vi "Ballistics_PBBA.vi"() -> ()   [LabVIEW 2012]
uses:
  <vilib>/Utility/NIReport.llb/NI_report.lvclass
  <vilib>/addons/database/NI_Database_API.lvlib
  <vilib>/addons/database/Connection.llb/Conn Execute.vi
  <vilib>/addons/database/Recordset.llb/Rec Destroy - Connection.vi
  <vilib>/Utility/config.llb/NI_LVConfig.lvlib
  <vilib>/Utility/config.llb/Write Key (I32).vi
  <vilib>/addons/database/Connection.llb/DB Tools Open Connec (String).vi
  <vilib>/addons/database/_DB Variant To Data/Database Variant To Data.xnode
  <vilib>/Analysis/NI_AALBase.lvlib
  <vilib>/Utility/config.llb/Write Key (String).vi
  <vilib>/Utility/NIReport.llb/Append Report Text (str wrap).vi
  <vilib>/Utility/NIReport.llb/Append Text Table to Report (wrap).vi
panel:
  in  "Case Constant 2":bool=TRUE
  in  "Case Constant 1":bool
  in  "Contact Shot Report":bool
  in  "message control":bool=TRUE
  in  "Stop Program":bool
  in  "switch":bool
  out "metric conversion":dbl=0.30480370641307 format="%.5f"
  out "number of completes":i32=3
  out "number of partials":i32=2
  in  "percent warning":dbl=1.0 format="%.2f"
  in  "old shots":T1(array[cluster]) {"Red Vel" format="%.2f"; "Energy Loss (J)" format="%.3e"; "Projectile Mass" format="%.4f"; "Corrected residual" format="%.2f"; "Uncorrected Residual" format="%.2f"; "Corrected Impact" format="%.2f"; "Uncorrected Impact" format="%.2f"; "Shot Angle" max=90 step=1; "SHOT STATUS" items=["Partial", "Complete"]; "IMPACT VELOCITY" min=0.0 max=10000.0 step=0.10000000149011612 format="%.1f"; "Barrel Temperature" format="%.1f"; "Powder Loading" format="%.4f"; "RESIDUAL  VELOCITY" min=0.0 max=10000.0 step=0.10000000149011612 format="%.1f"}
  in  "Version":dbl format="%.2f"
  out "Complete":dbl[](array[numeric]) format="%.2f"
  out "Partial":dbl[](array[numeric]) format="%.2f"
  in  "old drag":bool=TRUE
  out "impact/ID":u32=83886081 format="%.0x"
  out "residual/ID":u32=83951617 format="%.0x"
  out "Red/ID":u32=84017153 format="%.0x"
  out "correction coefficient":dbl format="%.8f"
  out "Corrected Residual":dbl format="%.2f"
  out "Corrected Impact":dbl=44.2924057714593 format="%.2f"
  out "plytypes":u16=1
  in  "Number of Ply Types":i32 min=0 max=20 step=1
  out "factor array":dbl[](array[numeric])=[0.0, 0.0, 0.0, 0.0, 0.0, 0.0, 0.0, 0.0, 0.0, 0.0, 0.0, 0.0, 0.0, 0.0, 0.0, 0.0, 0.0, 0.0252, 0.0, 0.0191, 0.0191, 0.0191, 0.0, 0.0, 0.0441, 0.0, 0.0, 0.0, 0.0, 0.0, 0.0, 0.0, 0.0425, 0.0, 0.0, 0.0131, 0.0, 0.0, 0.0, 0.018, 0.0, 0.0, 0.0, 0.0] format="%.4f"
  in  "reread":bool
  out "Weight Units":string
  out "Distance Units":string
  in  "Add Disclaimer":bool
  in  "Report":bool
  in  "RESET":bool
  in  "Save":bool
  in  "EXIT":bool
  in  "String":string="Ply Data Not Entered"
  in  "Enum":T2(ring)
  in  "Impact/Separation":dbl=4.0 format="%.2f"
  in  "Barrel to Screen Distance":dbl=7.8333 format="%.2f"
  in  "Impac/Target Dist":dbl=7.083333 format="%.2f"
  in  "Residual/Separation":dbl=4.0 format="%.2f"
  in  "Residual/Target Dist":dbl=7.083333 format="%.2f"
  out "Z.M.R.":dbl min=0.0 step=0.1 format="%.1f"
  in  "old threat":u32
  out "Shot Graph":cluster{i32[], sgl[]}[](graph)
  in  "Tab Control":T3(tab)
  out "String 2":string="Ballistic Test Program is now initializing.  This requires 30 seconds.  This message will be removed when the program is                ready to be used.                              NOTICE: After initialization, a test bullet must be fired daily to insure superior quality control"
  out "Corrected Redundant":dbl caption="REDUNDANT VELOCITY" min=0.0 max=10000.0 step=0.10000000149011612 format="%.1f"
  in  "backfacedia":dbl
  in  "backdepth":dbl
  out "% Difference":dbl=0.9916409839420799 format="%.1f"
  out "zmr 2":dbl caption="Z.M.R." format="%.1f"
  out "Pairs":i16 min=0 max=100 step=1
  out "Value":dbl format="%.1f"
  in  "Maximum Deviation":dbl=125.0 min=0.0 max=200.0 step=25.0 format="%.1f"
  in  "B.F.S (mm)":u16
  in  "N.I.J":u16(ring) items=["Not Tested", "PASS", "FAIL"]
  in  "Projectile Mass":dbl=7.1278801000000005 caption="Projectile Mass\n(grams)" min=0.0 step=1.0 format="%.4f"
  out "Residual":dbl=1.0 min=0.0 max=1.0 format="%.5f"
  out "Impact":dbl=1.0 min=0.0 max=1.0 format="%.5f"
  out "Shot":i32
  out "Panel":i32
  in  "Data Source":u16(ring)=2 items=["Simulated", "Radar", "Screens"]
  out "Database Connection":string
  in  "Report Path":path=path "c:/ballistic reports"
  in  "red/speed":dbl caption="REDUNDANT VELOCITY" min=0.0 max=1000000.0 step=0.10000000149011612 format="%.1f"
  out "CURRENT TIME / DATE":string
  in  "Current/residual/speed":dbl min=0.0 max=10000.0 step=0.10000000149011612 format="%.1f"
  in  "Current/sthotstatus":u16(ring) items=["Partial", "Complete"]
  in  "Current/impact/speed":dbl min=0.0 max=10000.0 step=0.10000000149011612 format="%.1f"
  in  "Shot Angle":u16 max=90 step=1
  out "BACKFACE DEPTH":dbl caption="BACKFACE\nDEPTH" min=0.0 max=200.0 step=5.0
  out "BACKFACE DIAMETER":dbl caption="BACKFACE\nDIAMETER" min=0.0 max=100.0 step=5.0
  in  "Drag Corrected":bool=TRUE
  in  "Reject shot":bool
  in  "Accept Data":bool
  in  "Powder Loading":dbl min=0.0 max=100.0 step=0.1 format="%.3f"
  in  "Shot Decription":string
  in  "Barrel Temp":dbl format="%.1f"
  out "SUBMIT DATE/TIME":string
  out "residual/speed":dbl caption="RESIDUAL  VELOCITY" min=0.0 max=10000.0 step=0.10000000149011612 format="%.1f"
  out "SHOT STATUS":u16(ring) items=["Partial", "Complete"]
  out "Impact/speed":dbl caption="IMPACT VELOCITY" min=0.0 max=10000.0 step=0.10000000149011612 format="%.1f"
  in  "Table of Shots":string[][](table) caption="Table"
  in  "RANGE RESET":bool
  in  "Tab Control 2":T4(tab)
  in  "Sample ID":string
  in  "Powder Type":u16(ring) items=["ACCURATE, NO. 2", "ACCURATE, NO.9", "Alliant 2400", "Alliant Herc. Bullseye", "Hercules", "Hi-Skor 700x", "Hi-Skor 800x", "IMR-4198", "IMR-4756", "IMR-4895", "International Clay's", "OTHER", "Power Pistol", "WINCHESTER-231", "WINCHESTER-296", "Winchester Ball"]
  in  "Test Comments":string
  in  "Test Conditions":u32(ring) items=["ACCELERATED AGEING", "CONDITIONED", "Cold", "Dry", "Hot 160 DEG. F", "MOTOR OIL", "WEAPON LUBRICANT", "Wet"]
  in  "ballistician":u16(ring) items=["n.a."]
  in  "Method":u16(ring) items=["CUSUM", "N.I.J.", "Quasi N.I.J.", "V(0)", "V(0) @ 1450", "V(0) @ 1500", "V(0) @ 1550", "V50", "VsVr"]
  in  "Room Temperature":i32
  in  "Room Humidity":i32
  in  "Panel Dimensions":u16(ring) items=["101/4\" X 113/4\"", "12X12", "12x15", "13\"X13\"", "15\" x 18\"", "15X16", "15x15", "15x15", "16X16", "18X18", "20X16", "24 x 24", "26X26", "7.5\" X 7.5\"", "8.5\" X 11\"", "CHEST PLATE", "HELMET", "NOT APPLICABLE", "VEST PANEL"]
  in  "Submitter":u16(ring) items=["other"]
  in  "Panel Backing":u16(ring) items=["Aluminum, 24 ga. (.020,.2024-T3) Witness Plate", "Clay (ROMA Plastilina # 1)", "None", "miscellaneous"]
  in  "Threat 2":u32(ring) items=["110-grain(non-toxic)NYLON, 38 SPECIAL, POLY-TUNGSTEN, 10\" SAMMI TEST BBL.", "115-GRAIN,9mm LUGER,REFERENCE ROUND,.38 caliber chamber,10\" TEST BBL.", "115-GRAIN,9mm LUGER,REFERENCE ROUND,10\", 9mm, TEST BBL.", "115-grain, 9 mm, HI-SHOK JHP, +P+ FEDERAL, 10\" SAMMI TEST BBL.", "115-grain, 9 mm, HI-SHOK JHP, +P+ FEDERAL, 5\" SAMMI TEST BBL.", "115-grain,9mm,SMJ,SVENKA-BULLET,CHILE,S.A. 10\"SAMMI TEST BBL.", "123-grain,7.62mm AK-47            7.62mm SAAMI test bbl.", "124-grain,9mm FMJ Rem.#23558, 10\".357cal.SAAMI test bbl.", "124-grain,9mm,FMJ,Rem.#23558, .38 caliber chamber, 10\"SAAMI test bbl.1/10\" TWIST", "124-grain,9mm,FMJ,Rem.#23558, 10\"SAAMI test bbl.", "124-grain,9mm,FMJ,Rem.#23558, 5\"SAAMI test bbl.", "127-grain,9mm,SXT/Blck Tln, +P+,Win.RA9SXT SAAMI test bbl.", "148 grain 7.62 x 51 mm M80 ball", "148-grain,7.62mm FMJ  M80     7.62mm SAAMI test bbl.", "158-grain,0.357, JSP, Rem.#22487 10\"SAAMI test bbl.", "158-grain,0.357, JSP,SPEER.#4217,10\"SAAMI test bbl.", "158-grain,WIN. 357 MAG, JHP REFERENCE ROUND, 10\" SAMMI TEST BBL.", "16-grain,  saboted RCC,.308cal.SAAMI test bbl.,DC", "166-grain,.30 cal. M2 AP, 7.62mm SAAMI test bbl.", "17-grain,sabot,STANAG 2920, FSP,.308 cal. SAMMI test bbl., DC", "17-grain,sabot.Type 1,FSP,.308cal.SAAMI test bbl.,DC", "17-grain,sabot.Type 2,FSP,.308cal.SAAMI test bbl.,DC", "180-grain,40 cal. S&W, 5\"SAMMI test bbl.", "180-grain,WIN. 308 POWER-POINT REFERENCE ROUND, 308 TEST BBL.", "2-grain, saboted RCC FSP,.223cal.SAAMI test bbl.,DC", "207 grain, FSP, 50 Cal", "240 grain,0.44, SWC Speer #4660 no gc,8\"SAAMI test bbl.", "240-grain,0.44, FMJ Speer #4459, 8\" SAMMI test bbl.", "240-grain,0.44, JSP Speer #4457       8\"SAAMI test bbl.", "240-grain,0.44, SJHP,  REM.  # 23592,   8\"SAAMI test bbl.", "240-grain,0.44, SWC PMC w/Gas Check   8\"SAAMI test bbl.", "240-grain,REM. .44 mag, JSP REFERENCE ROUND, 8\" SAMMI TEST BBL.", "4-grain, saboted RCC FSP ,.223cal.SAAMI test bbl.,DC", "44-grain, 0.30-cal FSP - no sabot", "44-grain, 0.30-cal FSP - no sabot", "44-grain,sabot.      FSP,.458cal.SAAMI test bbl.,DC", "45-grain,JHP(WIN), .223 cal. SAMMI test bbl.", "55-grain, 0.223 M-193 FMJ        .223cal.SAAMI test bbl.", "62-grain, 0.223 M-855 Green Tip  .223cal SAAMI test bbl.", "64-grain,sabot.  RCC,.458cal.SAAMI test bbl.,DC", "85-grain(non-toxic), 38 SPECIAL FRANGIBLE,WIN # RA38DF,10\" SAMMI TEST BBL.", "85-grain(non-toxic), 9mm FRANGIBLE +P+,WIN # RA9DF, 5\" SAMMI TEST BBL.", "85-grain(non-toxic), 9mm FRANGIBLE +P+,WIN # RA9DF,10\" SAMMI TEST BBL.", "85-grain, 7.62mm Tokarev(LEAD CORE-STEEL JACKET,1992)Tokarev SAAMI test bbl."]
  in  "Layers":T5(array[cluster])=[{"Ply Description"=0, "Layer Comments"="", "Number of Plies"=1}] {"Number of Plies" min=0 max=99 step=5; "Ply Description" items=["none"]}
  in  "Fabric Description":string
  out "Total Number of Layers":i32=1 caption="Total Number\nof Layers" min=0 max=100 step=5
  in  "Panel Technician":u16(ring) items=["Not Known", "POINT BLANK", "none"]
  in  "Weight of Panel":dbl format="%.4f"
  in  "Areal density text":string
  in  "Areal Density":dbl format="%.2f"
  in  "Thickness":dbl format="%.2f"
  in  "Manufacturer":u32(ring) caption="Mfr" items=["Point Blank-Marine Interceptor"]
  in  "Type":u16(ring) items=["none"]
  in  "Panel Type":u32(ring) items=["COMPOSITE ARMOR", "FABRIC ARMOR", "HELMET", "LG.RIGHT FRONT VEST PANEL", "N.A."]
  in  "Panel Stitch":u32(ring) items=["CAR ARMOR LAMINATE PANEL", "HARD PANEL", "N.A.", "TEST PANEL/CUSTOM STITCH", "TEST PANEL/NORMAL STITCH", "VEST PANEL/CUSTOM STITCH"]
  in  "Next Shot":bool
  in  "Delete Button":bool
  in  "SHOTS":T1(array[cluster]) {"Red Vel" format="%.1f"; "Energy Loss (J)" format="%.3e"; "Projectile Mass" min=0.0 step=1.0 format="%.4f"; "Corrected residual" format="%.2f"; "Uncorrected Residual" format="%.2f"; "Corrected Impact" format="%.2f"; "Uncorrected Impact" format="%.2f"; "Shot Angle" max=90 step=1; "SHOT STATUS" items=["Partial", "Complete"]; "IMPACT VELOCITY" min=0.0 max=10000.0 step=0.10000000149011612 format="%.1f"; "Barrel Temperature" format="%.1f"; "Powder Loading" format="%.4f"; "RESIDUAL  VELOCITY" min=0.0 max=10000.0 step=0.10000000149011612 format="%.1f"}
  out "Data retrieval":string="\nWORKING"
  out "Actual Number of \nRecords Returned":i32=1001
  in  "latest Date":string="1/1/2100"
  in  "DATE 3":string="1/1/2100"
  in  "DATE 2":string="1/1/1900"
  in  "velocity-loading":bool
  in  "Panel Search":bool
  in  "Earliest Date":string="1/1/1900"
  in  "?":u16=1001 min=1 max=10000 step=100
  out "v50 data 2":string[][](table)
  out "In Control":bool=TRUE caption="Control Status"
  in  "Threat":u16(ring) items=["115-GRAIN,9mm LUGER,REFERENCE ROUND,10\" .38 cal TEST BBL.", "158-grain,WIN. 357 MAG, JHP REFERENCE ROUND, 10\" SAMMI TEST BBL.", "180-grain,WIN. 308 POWER-POINT REFERENCE ROUND, 308 TEST BBL.", "240-grain,REM. .44 mag, JSP REFERENCE ROUND, 8\" SAMMI TEST BBL."]
  in  "Powder":string="bul"
  out "St. Deviation":dbl=31.606020957071 format="%.1f"
  out "Latest Velocity":dbl=1314.9 format="%.1f"
  out "Average Velocity":dbl=1297.749514563107 format="%.1f"
  out "Previous V50 Data":cluster{dbl, dbl, dbl[][]}(graph)={0.0, 1.0, []}
  in  "Threat":string
  out "Velocity  versus Loading":cluster{dbl[], dbl[]}(graph)
  out "v50 data":string[][](table)
  out "Device S/N":string
  in  "DAQ Card":i16=1
  in  "Impact Timer":i16 min=0 max=3 step=1
  in  "Redundant Timer":i16=1 min=0 max=3 step=1
  in  "Residual  Timer":i16=2 min=0 max=3 step=1
  # "NOTE:Number of  plies must be entered in FABRIC INFORMATION to enable saving"
  # "yes"
  # "No"
  # "Yes"
  # "No"
  # "Point Blank Body Armor"
  # "Current Shot Data"
  # "Last Assigned  Number"
  # "V50"
  # "Correction Factor"
  # "Edit any non-date field by placing cursor in field. \n\nProperties not listed are controlled by the current shot, test description or Fabric information.  If the entry is changed for the current shot, then all previous shots are changed"
  # "CUSUM HISTORY"
  # "SHOT DATA"
  # "Max Records Returned\n (up to 10,000)"
  # "Date Range"
  # "(Form: 1/25/2000)"
  # "Date Range"
  # "Begin date"
  # "End Date"
  # "(Form: 1/25/2000)"
  # "End Date"
  # "Begin Date"
  # "Point Blank Body Armor\nBallistics Test Station\n\nVersion 1.00 BETA\n\nSeptember 2006"
  # "For technical support contact\n\nPat Fitzgerald or Mark Hartsky\n\nDuPont Company"
  # "This program is beta software and is based on the Ballistics Test Version 2005 developed internally by DuPont as a research tool for their Spruance Plant Ballistics Lab in Richmond, VA.  \n\nThis new version, adapted for use by DHB Point Blank Body Armor, is modified from its original design and does not depend on safety interlock systems to enable operation of a ballistics test.\n\nDuPont makes no warranties and assumes no liabilities in connection with any use of this program."
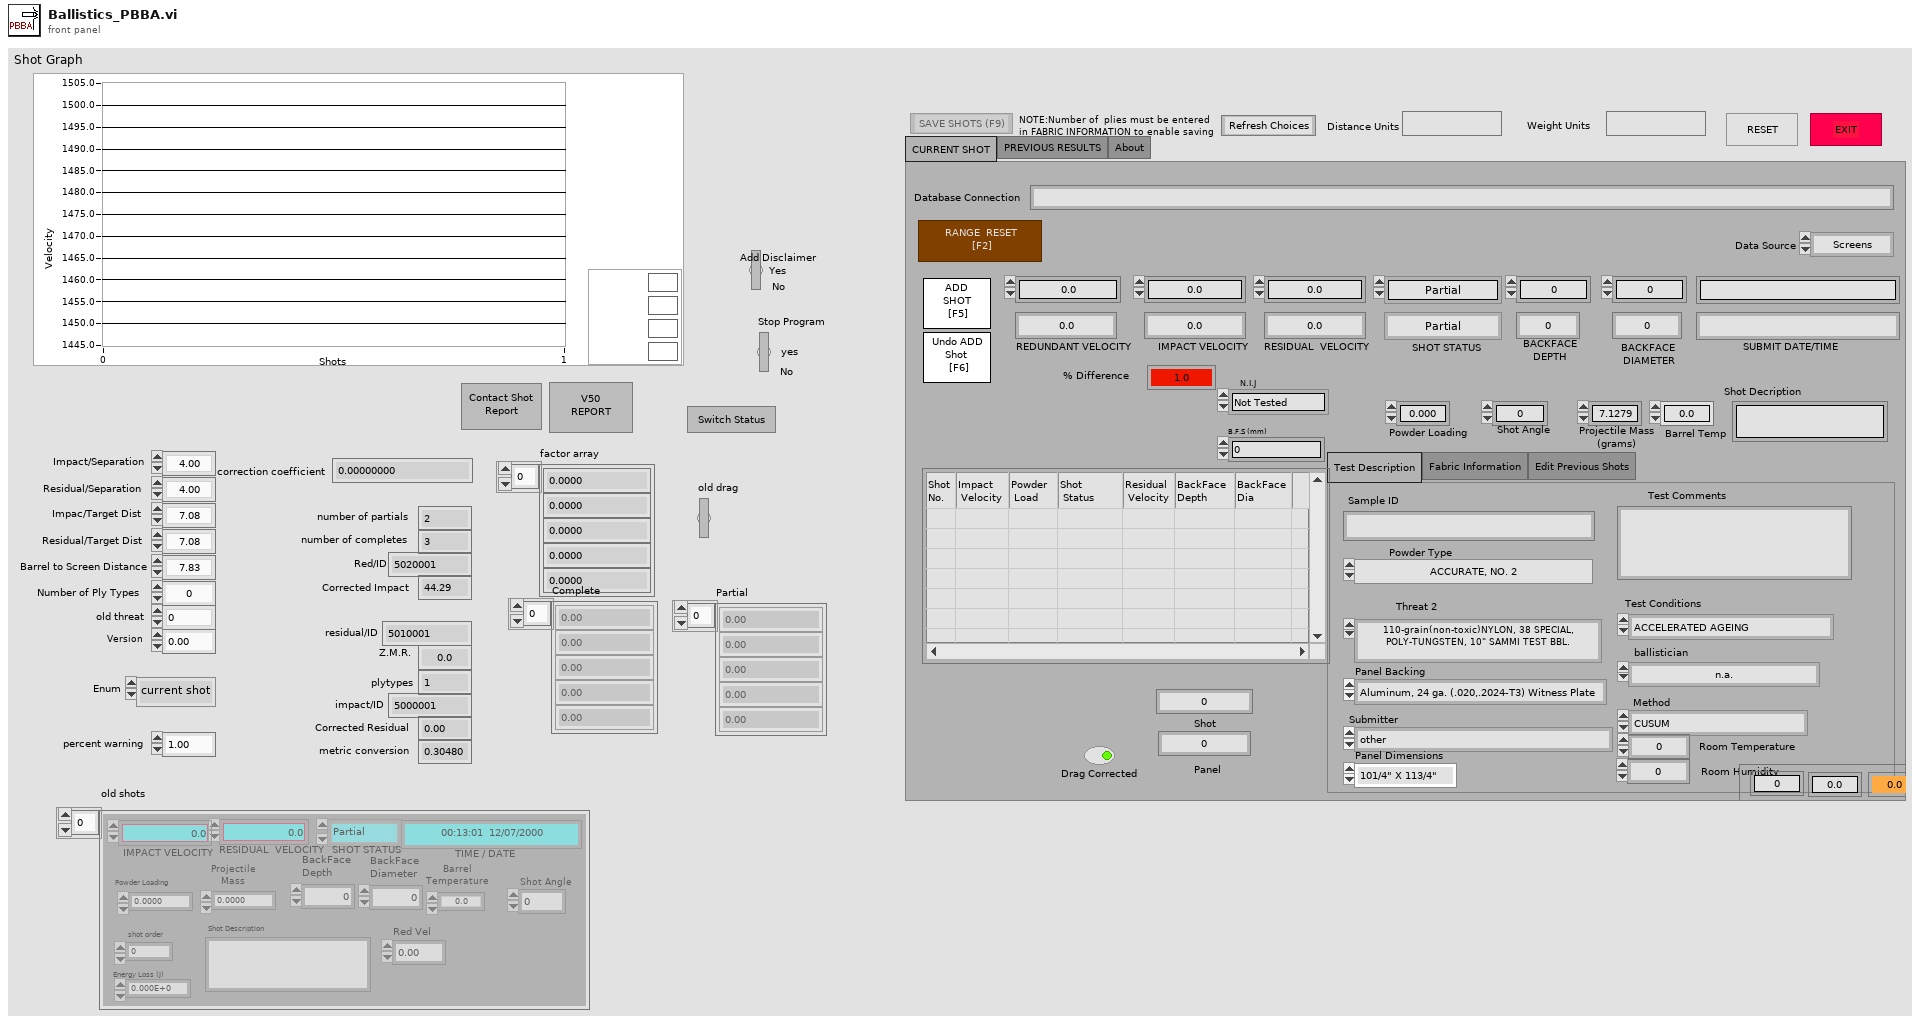
[diagram p1: front panel]
types:
  T1 = cluster{"IMPACT VELOCITY":dbl, "RESIDUAL  VELOCITY ":dbl, "Shot Description":string, "Powder Loading ":dbl, "Barrel Temperature":dbl, "TIME / DATE":string, "shot order":i32, "SHOT STATUS":u16, "Shot Angle":u16, "Uncorrected Impact":dbl, "Corrected Impact":dbl, "Uncorrected Residual":dbl, "Corrected residual":dbl, "Projectile Mass":dbl, "usedv50":bool, "Energy Loss (J)":sgl, "BackFace\nDepth":dbl, "BackFace\nDiameter":dbl, "Red Vel":dbl}[]
  T2 = enum16{"current shot", "previous shots", "controls", "target data"}
  T3 = enum32{"CURRENT SHOT", "PREVIOUS RESULTS", "About"}
  T4 = enum32{"Test Description", "Fabric Information", "Edit Previous Shots"}
  T5 = cluster{"Ply Description":u16, "Layer Comments":string, "Number of Plies":i32}[]
  T6 = cluster{"impactCntrID":u32, "redundantCntrID":u32, "residualCntrID":u32}
  T7 = enum32{"existing file", "new file", "new or existing file", "existing dir", "new dir", "new or existing dir", "existing file (use LLBs)", "new file (use LLBs)", "new or existing file (use LLBs)", "new or existing file or directory (use LLBs)"}
  T8 = typedef "NI_LVConfig.lvlib/Config Data RefNum.ctl" = refnum<k1>
  T9 = cluster{"Charset (-1)":i16, "Weight (-1)":i16, "Name":string, "Size":string}
  T10 = cluster{"Italic":enum16{"Italic Unchanged", "Italic On", "Italic Off"}, "Strike Through":enum16{"Strike Through Unchanged", "Strike Through On", "Strike Through Off"}, "Underline":enum16{"Underline Unchanged", "Underline On", "Underline Off"}, "Bold":enum16{"Bold Unchanged", "Bold On", "Bold Off"}}
  T11 = cluster{"IMPACT VELOCITY":dbl, "RESIDUAL  VELOCITY ":dbl, "Shot Description":string, "Powder Loading ":dbl, "Barrel Temperature":dbl, "TIME / DATE":string, "shot order":i32, "SHOT STATUS":u16, "Shot Angle":u16, "Uncorrected Impact":dbl, "Corrected Impact":dbl, "Uncorrected Residual":dbl, "Corrected residual":dbl, "Projectile Mass":dbl, "usedv50":bool, "Energy Loss (J)":sgl, "BackFace\nDepth":dbl, "BackFace\nDiameter":dbl, "Red Vel":dbl}
  T12 = typedef "NI_Database_API.lvlib/Conn ObjectReference.ctl" = refnum<k1>
  T13 = typedef "NI_Database_API.lvlib/Rec ObjectReference.ctl" = refnum<k1>
  T14 = enum16{"Standard Report", "HTML", "Word", "Excel"}
  T15 = cluster{"task ID out":u32, "task ID out":u32, "task ID out":u32}
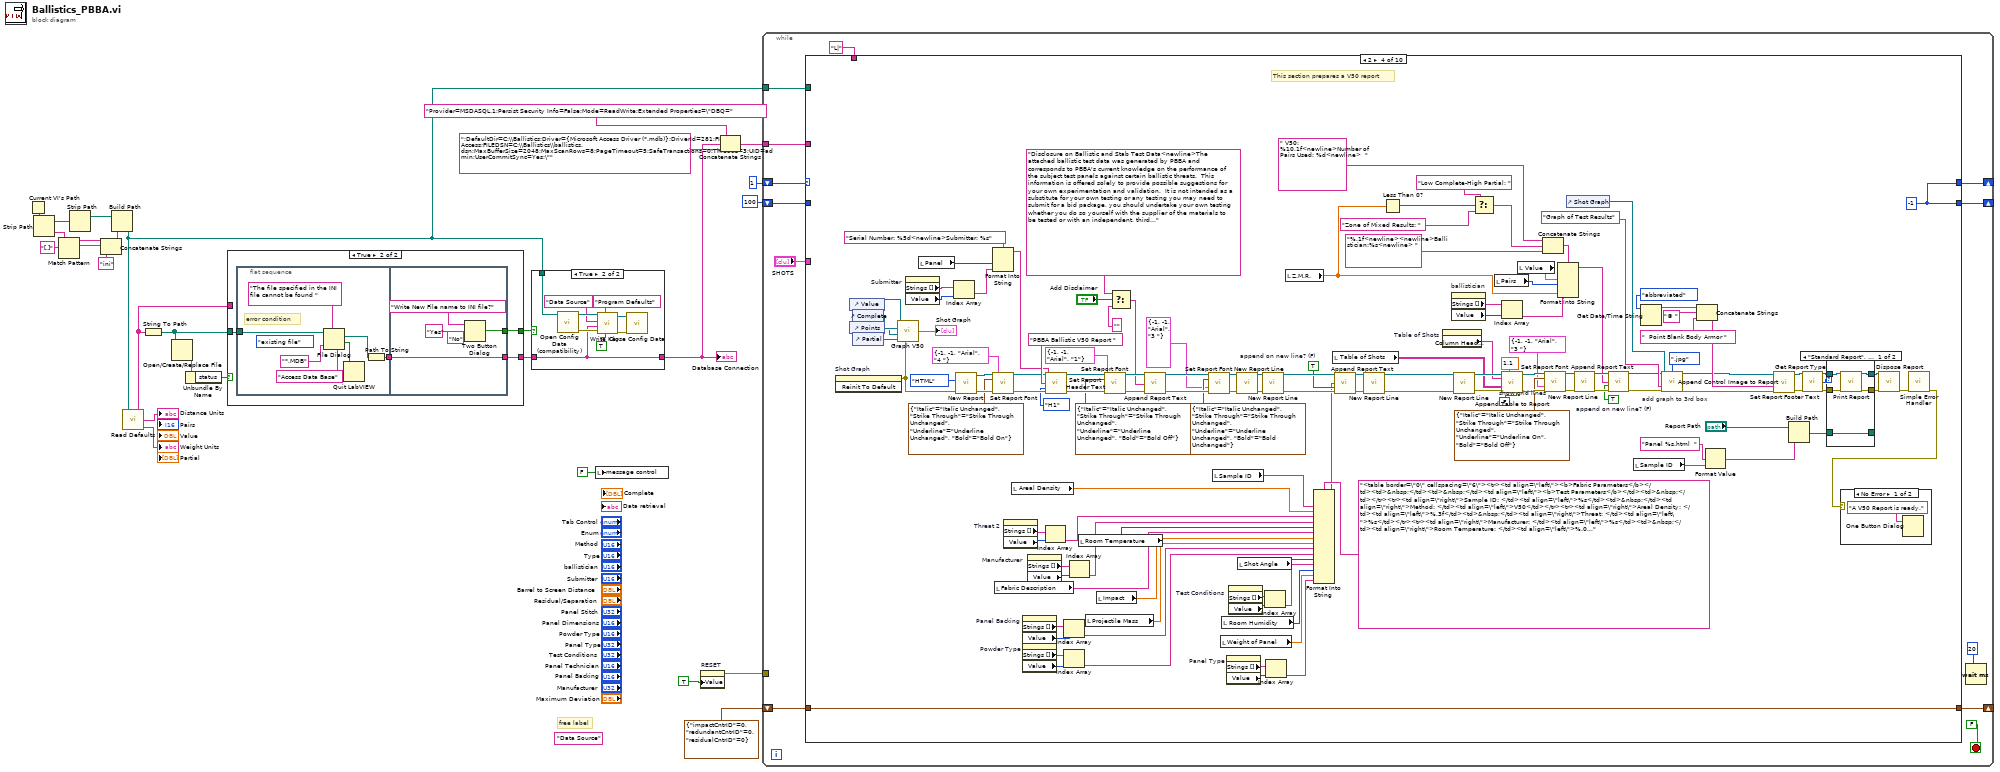
[diagram p0: block diagram]
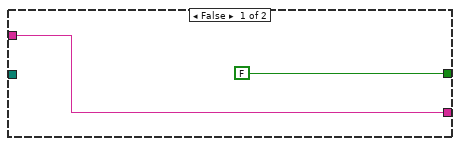
[diagram p3: hidden frame]
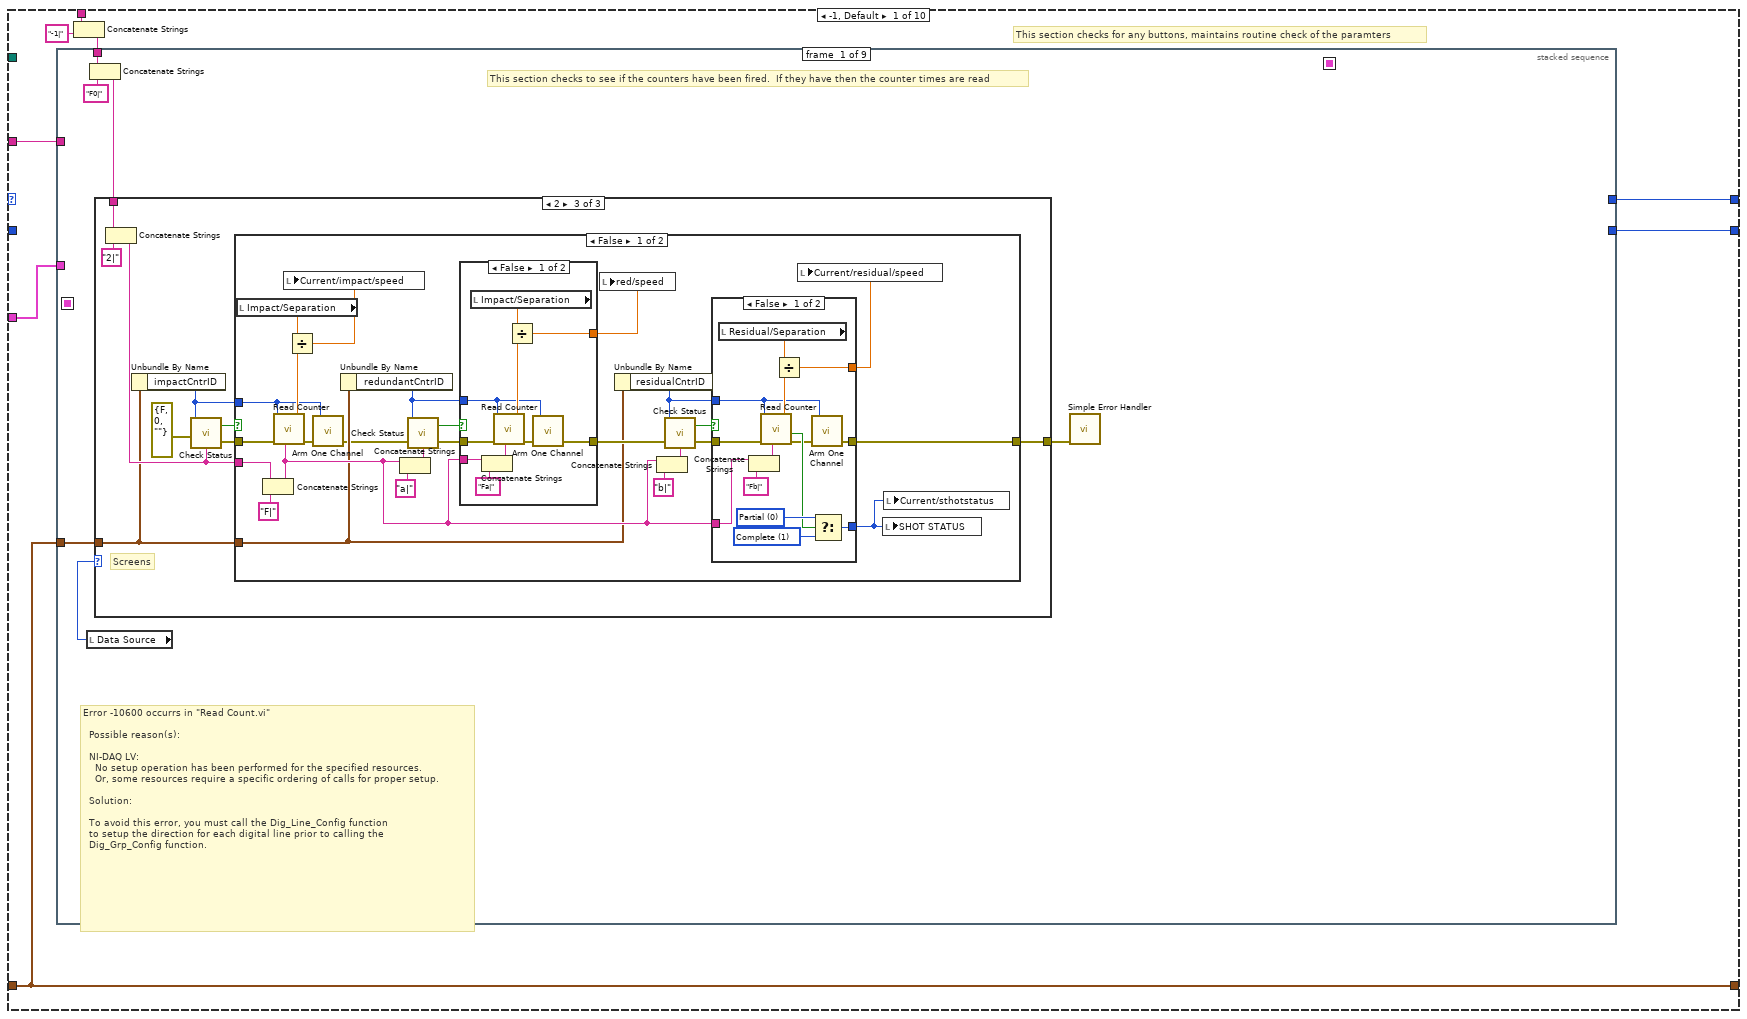
[diagram p4: hidden frame]
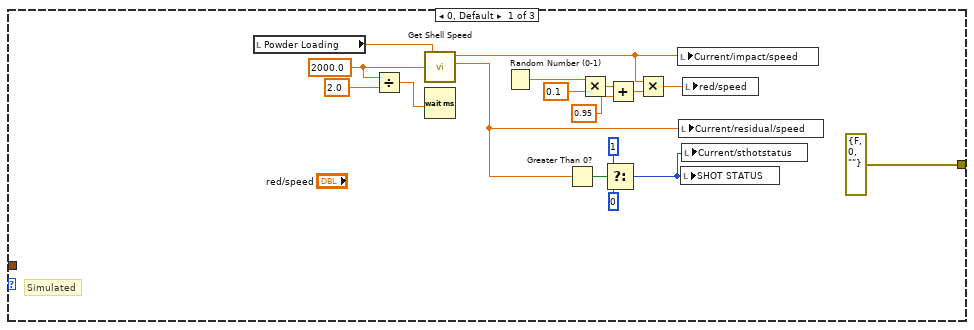
[diagram p5: hidden frame]
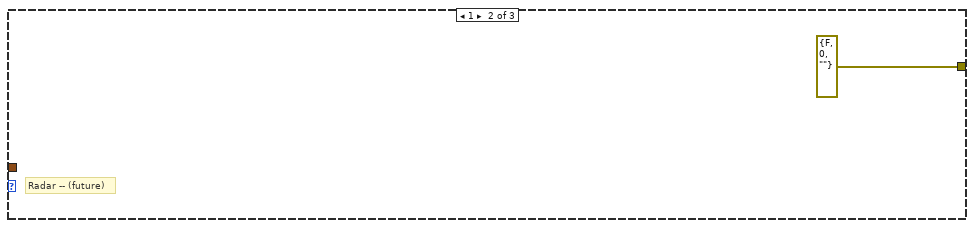
[diagram p6: hidden frame]
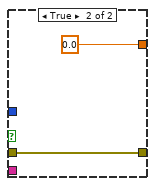
[diagram p7: hidden frame]
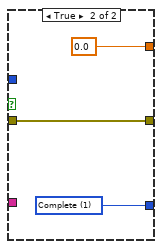
[diagram p8: hidden frame]
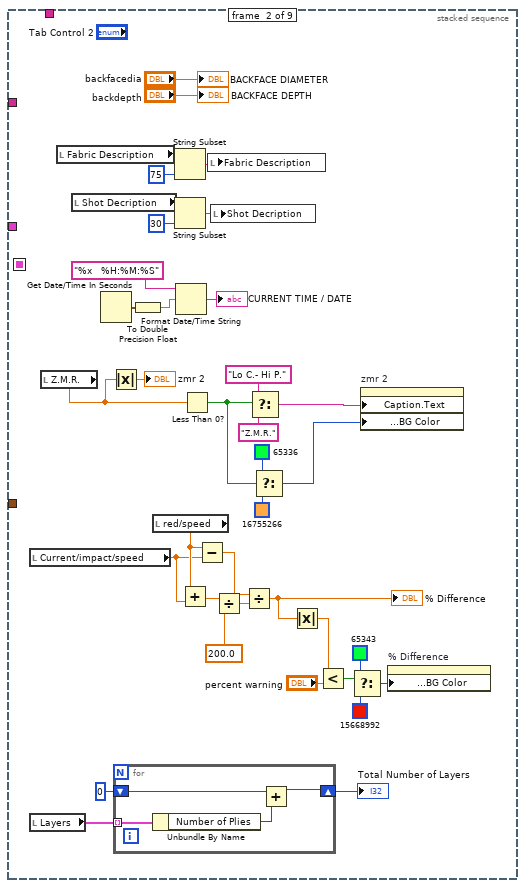
[diagram p10: hidden frame]
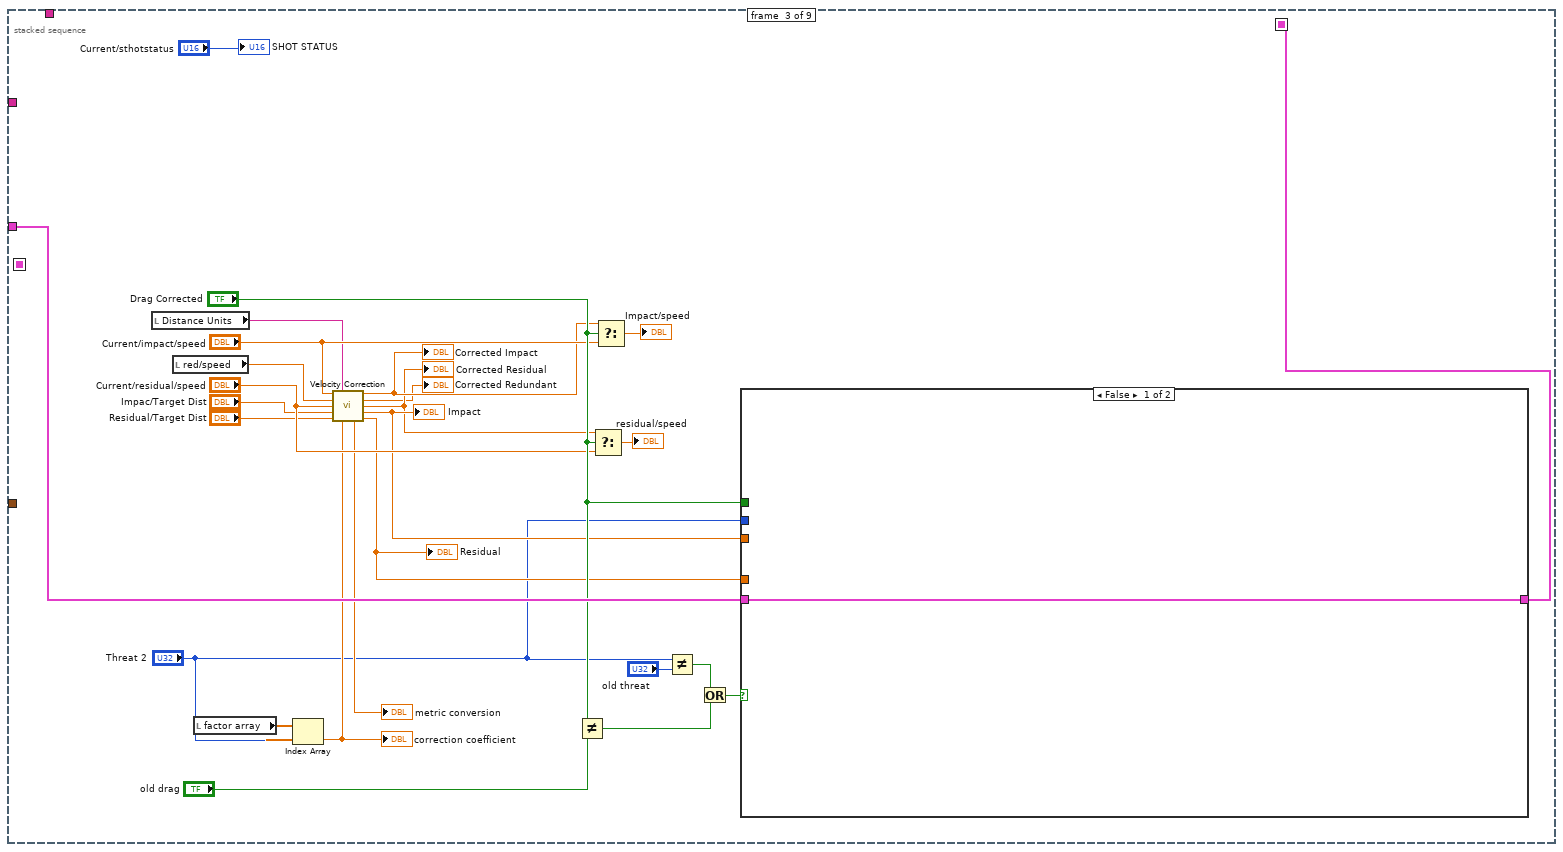
[diagram p11: hidden frame]
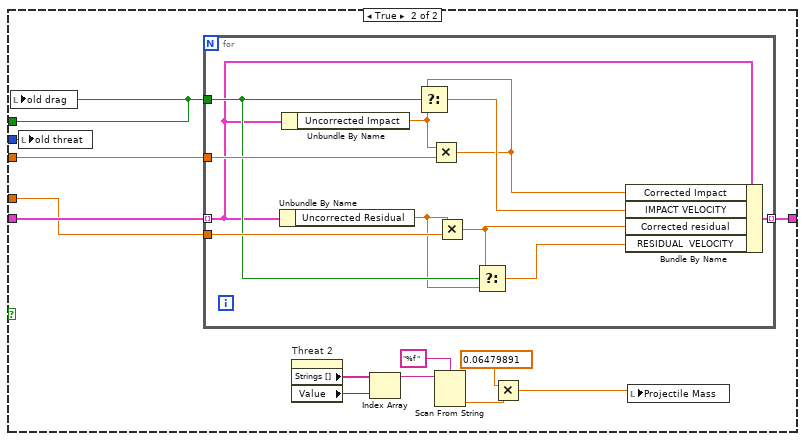
[diagram p12: hidden frame]
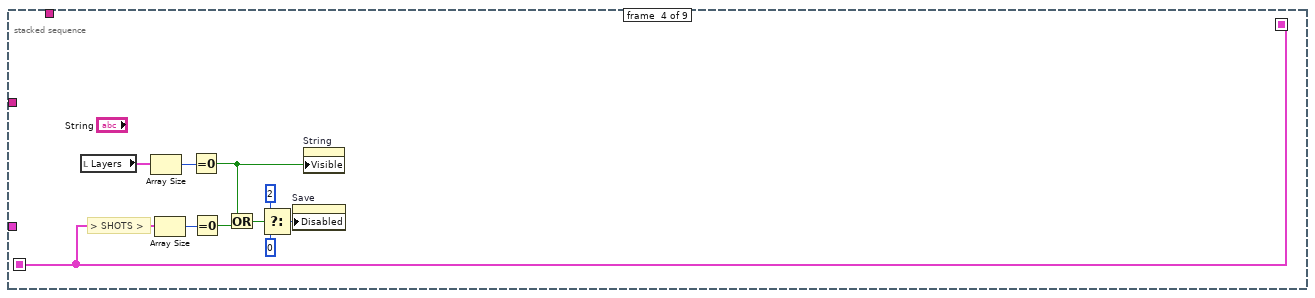
[diagram p13: hidden frame]
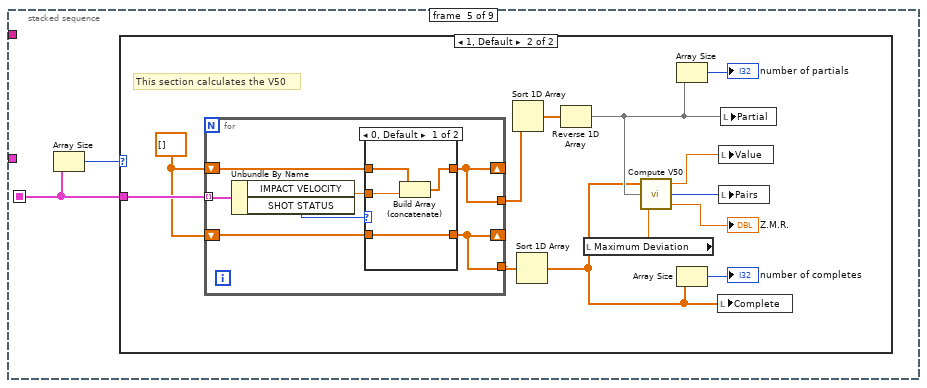
[diagram p14: hidden frame]
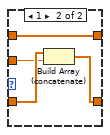
[diagram p16: hidden frame]
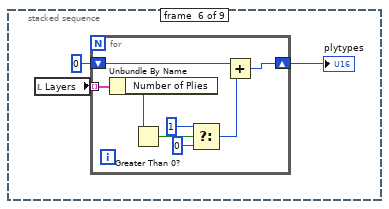
[diagram p17: hidden frame]
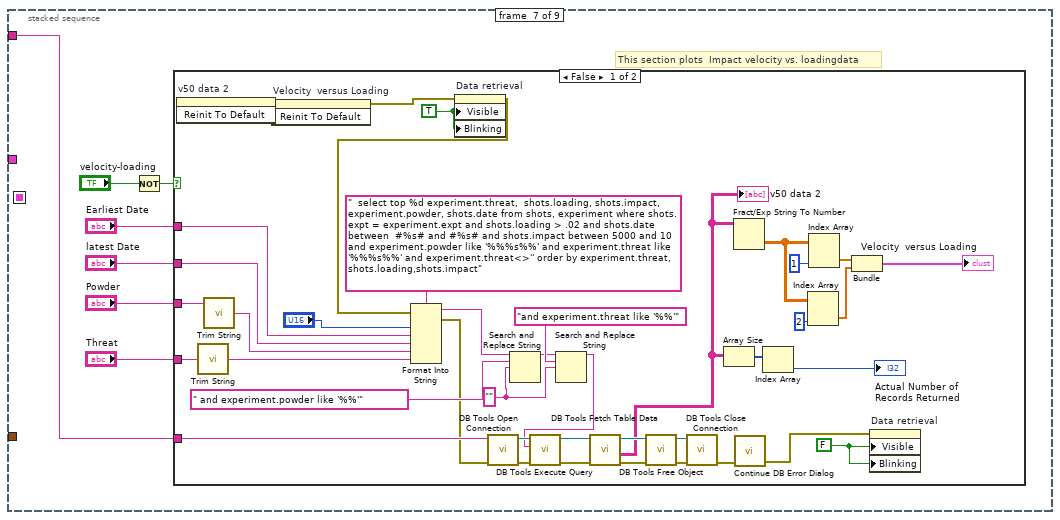
[diagram p18: hidden frame]
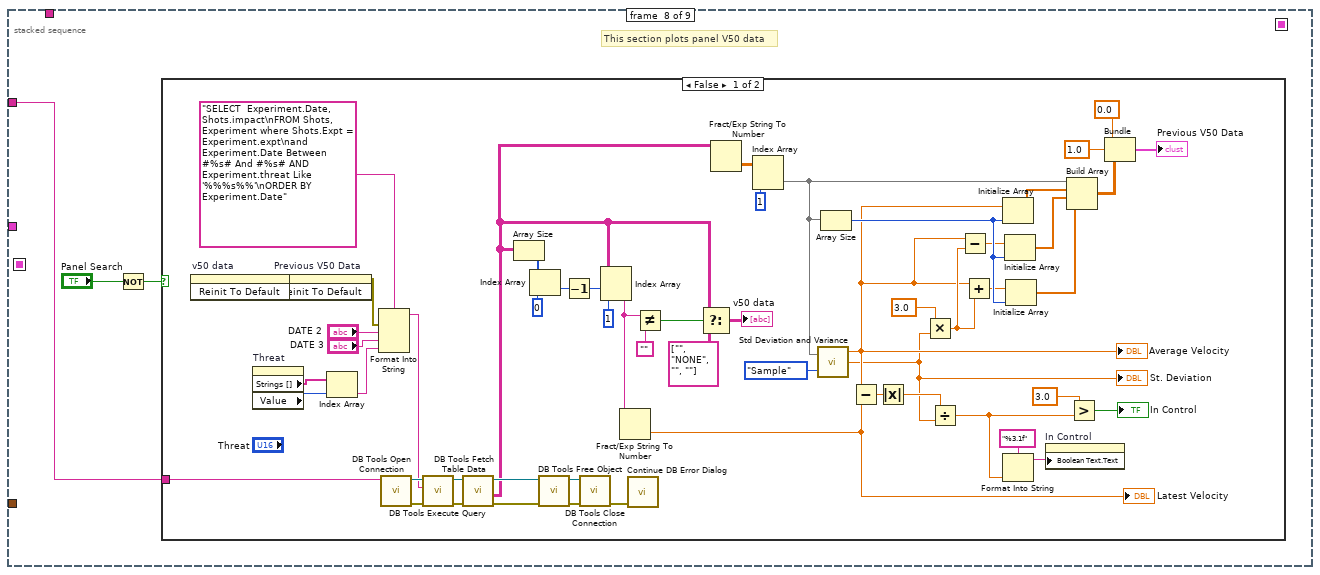
[diagram p20: hidden frame]
diagram:
  (unwired) "Data Source" ("key")
  # "free label"
  n1 = Current VI's Path() -> (path=w25:path)
  n2 = Strip Path(path=w25) -> (stripped path=w24:path, name=w22:string)
  n3 = Match Pattern(string=w22, regular expression="[.]") -> (before substring=w19:string, match substring=w18:string)  [unwired: 1 in, 2 out]
  n4 = Strip Path(path=w24) -> (stripped path=w17:path)  [unwired: 1 out]
  n5 = Concatenate Strings(w19, w18, "ini" ("string")) -> (w21:string)
  n6 = Build Path(base path=w17, name or relative path=w21) -> (appended path=w2:path)
  n7 = call "Read Defaults.vi"("appended path"=w2) -> ("value"=w10:string, "String"=→"Distance Units":string, "String 2"=→"Weight Units":string)
  n8 = String To Path(string=w10) -> (path=w13:path)
  n9 = Open/Create/Replace File(file path (use dialog)=w13) -> (error out=w14:errorcluster)  [unwired: 5 in, 2 out]
  n10 = Unbundle By Name(w14) -> ("status"=w3:bool)
  n11 = case shown="True" w3 {
    tunnel: w10 -> [w30 _]
    tunnel: [w30 w31] -> w9
    tunnel: w13 -> [_ w34]
    tunnel: [FALSE ("T button?") w32] -> w8
    frame False {
    }
    frame True {
      n12 = flat-sequence {
        tunnel: w34 -> [w41]
        tunnel: [w40] -> w33
        tunnel: [w42] -> w31
        tunnel: w33 -> [w42]
        tunnel: [w43] -> w32
        frame #0 {
          (unwired) T7."existing file" ("select mode (2)")
          # "error condition"
          n13 = File Dialog(4:"Access Data Base" ("pattern label"), 6:"*.MDB" ("pattern"), 7:"The file specified in the INI file cannot be found " ("prompt"), 11:w41) -> (1:w35:bool, 3:w38:path)  [unwired: 3 in, 2 out]
          n14 = Quit LabVIEW(quit? (T)=w35) -> ()
          n15 = Path To String(path=w38) -> (string=w40:string)
        }
        frame #1 {
          n16 = Two Button Dialog(message="Write New File name to INI file?", 1:"No" ("F button name (\"Cancel\")"), 2:"Yes" ("T button name (\"OK\")")) -> (T button?=w43:bool)
        }
      }
    }
  }
  n17 = case shown="True" w8 {
    tunnel: w9 -> [w47 w52]
    tunnel: [w47 w52] -> w6
    tunnel: w2 -> [_ w48]
    frame False {
    }
    frame True {
      n18 = call <vilib>:"Open Config Data (compatibility).vi"("configuration file path"=w48) -> ("error out"=w53:errorcluster, "refnum"=w56:T8)  [unwired: 8 in, 1 out]
      n19 = call-poly <vilib>:"Write Key.vi"("write raw string? (F)"=TRUE, "section"="Program Defaults", "error in (no error)"=w53, "value"=w52, "key"="Data Source", "refnum"=w56) -> ("error out"=w51:errorcluster, "refnum out"=w50:T8)  [unwired: 3 in, 1 out]
      n20 = call <vilib>:"Close Config Data.vi"("error in (no error)"=w51, "refnum"=w50) -> ()  [unwired: 8 in, 2 out]
    }
  }
  "Database Connection" <- w6
  n21 = local write "message control"(FALSE) -> ()
  n22 = property on="RESET" class="Bool (strict)"("Value"=TRUE ("RESET")) -> (error out=w4:errorcluster)  [unwired: 2 in, 1 out]
  n23 = Concatenate Strings("Provider=MSDASQL.1;Persist Security Info=False;Mode=ReadWrite;Extended Properties=\"DBQ=", w6, ";DefaultDir=C:\\Ballistics;Driver={Microsoft Access Driver (*.mdb)};DriverId=281;FIL=MS Access;FILEDSN=C:\\Ballistics\\ballistics.dsn;MaxBufferSize=2048;MaxScanRows=8;PageTimeout=5;SafeTransactions=0;Threads=3;UID=admin;UserCommitSync=Yes;\"") -> (w7:string)
  n24 = while {
    shift-left: 100 -> [w64]
    shift-right: [w65] -> _
    shift-left: 1 ("index of element") -> [w68]
    shift-right: [w66] -> _
    tunnel: w2 -> [w61]
    tunnel: w7 -> [w60]
    tunnel: w4 -> [_]
    shift-right: [w58] -> _
    shift-left: T6 {"impactCntrID"=0, "redundantCntrID"=0, "residualCntrID"=0} -> [w57]
    stop <- FALSE stop-if-true
    n25 = case shown="2" w68 {
      tunnel: [w74 w495 w500 w798 w817 w1008 w1046 w1054 w1098 w1221] -> w66
      tunnel: [w75 w495 w500 w798 w816 w1008 w1046 w1054 w1098 w1221] -> w65
      tunnel: w64 -> [_ _ w503 _ _ _ _ _ _ _]
      tunnel: "SHOTS" -> [w76 _ _ _ w815 w998 w1028 _ w1096 _]
      tunnel: w61 -> [_ _ w502 _ w813 _ _ _ _ _]
      tunnel: w60 -> [w73 _ w501 _ w812 _ _ _ _ _]
      tunnel: "L|" -> [w72 _ _ _ _ _ _ w1050 _ _]
      tunnel: [w69 w494 w499 w667 w810 w996 w1011 w1048 w1093 w1149] -> w58
      tunnel: w57 -> [w69 w494 w499 w667 w810 w996 w1011 w1047 w1093 w1149]
      frame -1, Default {
        # "This section checks for any buttons, maintains routine check of the paramters"
        n26 = Concatenate Strings(w72, "-1|") -> (w70:string)
        n27 = stacked-sequence {
          seq-local: [_ _ _ w258 _ _ _ _ _] -> [_ _ _ _ w269 _ _ _ w424]
          seq-local: [_ _ w221 _ _ _ _ _ _] -> [_ _ _ w258 _ _ _ _ _]
          tunnel: w76 -> [_ _ w227 _ _ _ _ _ _]
          tunnel: [_ _ _ _ _ _ _ _ w429] -> w74
          tunnel: [_ _ _ _ _ _ _ _ -1] -> w75
          tunnel: w73 -> [_ _ _ _ _ _ w309 w356 _]
          tunnel: w70 -> [w80 _ _ _ _ _ _ _ _]
          tunnel: w69 -> [w77 _ _ _ _ _ _ _ _]
          frame #0 {
            # "Error -10600 occurrs in \"Read Count.vi\"\n\n  Possible reason(s):\n\n  NI-DAQ LV:\n    No setup operation has been performed for the specified resources.\n    Or, some resources require a specific ordering of calls for proper setup.  \n\n  Solution: \n\n  To avoid this error, you must call the Dig_Line_Config function \n  to setup the direction for each digital line prior to calling the \n  Dig_Grp_Config function."
            # "This section checks to see if the counters have been fired.  If they have then the counter times are read"
            n28 = local read "Data Source"() -> (w82:u16)
            n29 = Concatenate Strings(w80, "F0|") -> (w78:string)
            n30 = case shown="2" w82 {
              tunnel: [errorcluster {"status"=FALSE, "code"=0, "source"=""} ("error out") errorcluster {"status"=FALSE, "code"=0, "source"=""} ("error out") w109] -> w81
              tunnel: w78 -> [_ _ w105]
              tunnel: w77 -> [_ _ w101]
              frame 0, Default {
                w98 = 2000.0 ("v50")
                # "Simulated"
                n31 = local read "Powder Loading"() -> (w97:dbl)
                n32 = Divide(x=w98, y=2.0 ("v50")) -> (x/y=w99:dbl)
                n33 = call "Get Shell Speed.vi"("loading"=w97, "v50"=w98) -> ("impact"=w85:sgl, "residual"=w91:sgl)  [unwired: 2 in, 1 out]
                n34 = Wait (ms)(milliseconds to wait=w99) -> ()  [unwired: 1 out]
                n35 = Random Number (0-1)() -> (number: 0 to 1=w89:dbl)
                n36 = Greater Than 0?(x=w91) -> (x > 0?=w94:bool)
                n37 = Multiply(x=w89, y=0.1) -> (x*y=w88:dbl)
                n38 = Select(t=u16 1, s=w94, f=u16 0) -> (s? t:f=w92:u16)
                n39 = Add(x=w88, y=0.95) -> (x+y=w86:dbl)
                n40 = Multiply(x=w85, y=w86) -> (x*y=w84:dbl)
                n41 = local write "Current/impact/speed"(w85) -> ()
                n42 = local write "Current/residual/speed"(w91) -> ()
                n43 = local write "SHOT STATUS"(w92) -> ()
                n44 = local write "Current/sthotstatus"(w92) -> ()
                n45 = local write "red/speed"(w84) -> ()
              }
              frame 1 {
                # "Radar -- (future)"
              }
              frame 2 {
                # "Screens"
                n46 = Concatenate Strings(w105, "2|") -> (w104:string)
                n47 = Unbundle By Name(w101) -> ("impactCntrID"=w102:u32)
                n48 = call "Check Status.vi"("error in (no error)"=errorcluster {"status"=FALSE, "code"=0, "source"=""}, "TL Calling Location"=w104, "Task ID"=w102) -> ("error out"=w107:errorcluster, "Armed?"=w103:bool)  [unwired: 1 in]
                n49 = case shown="False" w103 {
                  tunnel: w107 -> [w127 w165]
                  tunnel: [w128 w165] -> w109
                  tunnel: w102 -> [w110 _]
                  tunnel: w104 -> [w123 _]
                  tunnel: w101 -> [w113 _]
                  frame False {
                    n50 = local read "Impact/Separation"() -> (w132:dbl)
                    n51 = Concatenate Strings(w123, "F|") -> (w118:string)
                    n52 = call "Read Counter.vi"("TL Calling Location"=w118, "error In"=w127, "TASK ID"=w110) -> ("error out"=w112:errorcluster, "time (secs)"=w135:sgl)  [unwired: 3 in, 2 out]
                    n53 = Divide(x=w132, y=w135) -> (x/y=w130:dbl)
                    n54 = local write "Current/impact/speed"(w130) -> ()
                    n55 = call "Arm One Channel.vi"("error IN"=w112, "task ID IN"=w110) -> ("error out"=w111:errorcluster)  [unwired: 2 in, 1 out]
                    n56 = Unbundle By Name(w113) -> ("redundantCntrID"=w115:u32)
                    n57 = Concatenate Strings(w118, "a|") -> (w121:string)
                    n58 = call "Check Status.vi"("error in (no error)"=w111, "TL Calling Location"=w121, "Task ID"=w115) -> ("error out"=w126:errorcluster, "Armed?"=w117:bool)  [unwired: 1 in]
                    n59 = case shown="False" w117 {
                      tunnel: [w143 0.0] -> w134
                      tunnel: w126 -> [w142 w147]
                      tunnel: [w137 w147] -> w129
                      tunnel: w115 -> [w136 _]
                      tunnel: w118 -> [w140 _]
                      frame False {
                        n60 = local read "Impact/Separation"() -> (w144:dbl)
                        n61 = Concatenate Strings(w140, "Fa|") -> (w139:string)
                        n62 = call "Read Counter.vi"("TL Calling Location"=w139, "error In"=w142, "TASK ID"=w136) -> ("error out"=w138:errorcluster, "time (secs)"=w145:sgl)  [unwired: 3 in, 2 out]
                        n63 = Divide(x=w144, y=w145) -> (x/y=w143:dbl)
                        n64 = call "Arm One Channel.vi"("error IN"=w138, "task ID IN"=w136) -> ("error out"=w137:errorcluster)  [unwired: 2 in, 1 out]
                      }
                      frame True {
                      }
                    }
                    n65 = local write "red/speed"(w134) -> ()
                    n66 = Unbundle By Name(w113) -> ("residualCntrID"=w114:u32)
                    n67 = Concatenate Strings(w118, "b|") -> (w119:string)
                    n68 = call "Check Status.vi"("error in (no error)"=w129, "TL Calling Location"=w119, "Task ID"=w114) -> ("error out"=w125:errorcluster, "Armed?"=w116:bool)  [unwired: 1 in]
                    n69 = case shown="False" w116 {
                      tunnel: w125 -> [w154 w163]
                      tunnel: [w159 w164] -> w133
                      tunnel: w114 -> [w149 _]
                      tunnel: [w148 w163] -> w128
                      tunnel: [w156 0.0] -> w131
                      tunnel: w118 -> [w151 _]
                      frame False {
                        w160 = u16 1 items=["Partial", "Complete"] ("SHOT STATUS")
                        w161 = u16 0 items=["Partial", "Complete"] ("SHOT STATUS")
                        n70 = local read "Residual/Separation"() -> (w155:dbl)
                        n71 = Concatenate Strings(w151, "Fb|") -> (w152:string)
                        n72 = call "Read Counter.vi"("TL Calling Location"=w152, "error In"=w154, "TASK ID"=w149) -> ("error out"=w150:errorcluster, "counter overflow?"=w157:bool, "time (secs)"=w158:sgl)  [unwired: 3 in, 1 out]
                        n73 = Divide(x=w155, y=w158) -> (x/y=w156:dbl)
                        n74 = call "Arm One Channel.vi"("error IN"=w150, "task ID IN"=w149) -> ("error out"=w148:errorcluster)  [unwired: 2 in, 1 out]
                        n75 = Select(t=w161, s=w157, f=w160) -> (s? t:f=w159:u16)
                      }
                      frame True {
                        (unwired) 0.0
                        w164 = u16 1 items=["Partial", "Complete"] ("SHOT STATUS")
                      }
                    }
                    n76 = local write "Current/residual/speed"(w131) -> ()
                    n77 = local write "SHOT STATUS"(w133) -> ()
                    n78 = local write "Current/sthotstatus"(w133) -> ()
                  }
                  frame True {
                  }
                }
              }
            }
            n79 = call <vilib>:"Simple Error Handler.vi"("error in (no error)"=w81) -> ()  [unwired: 4 in, 5 out]
          }
          frame #1 {
            n80 = local read "Current/impact/speed"() -> (w185:dbl)
            n81 = local read "Layers"() -> (w201:T5)
            n82 = local read "Z.M.R."() -> (w188:dbl)
            n83 = local read "Fabric Description"() -> (w172:string)
            n84 = local read "Shot Decription"() -> (w169:string)
            n85 = Get Date/Time In Seconds() -> (seconds since 1Jan1904=w166:timestamp)
            n86 = Absolute Value(x=w188) -> (abs(x)=→"zmr 2":dbl)
            n87 = for {
              tunnel: w201 -> [w203] mode=indexing
              shift-right: [w205] -> w199
              shift-left: 0 -> [w204]
              n88 = Unbundle By Name(w203) -> ("Number of Plies"=w206:i32)
              n89 = Add(x=w204, y=w206) -> (x+y=w205:i32)
            }
            "Total Number of Layers" <- w199
            n90 = To Double Precision Float(number=w166) -> (double precision float=w196:dbl)
            n91 = local read "red/speed"() -> (w186:dbl)
            n92 = String Subset(string=w172, length (rest)=75 ("length (rest)")) -> (substring=w171:string)  [unwired: 1 in]
            n93 = String Subset(string=w169, length (rest)=30 ("length (rest)")) -> (substring=w167:string)  [unwired: 1 in]
            n94 = Format Date/Time String(time format string (%c)="%x   %H:%M:%S", seconds (now)=w196) -> (date/time string=→"CURRENT TIME / DATE":string)  [unwired: 1 in]
            n95 = Add(x=w186, y=w185) -> (x+y=w184:dbl)
            n96 = Less Than 0?(x=w188) -> (x < 0?=w194:bool)
            n97 = Subtract(x=w186, y=w185) -> (x-y=w187:dbl)
            n98 = local write "Fabric Description"(w171) -> ()
            n99 = local write "Shot Decription"(w167) -> ()
            n100 = Divide(x=w184, y=200.0) -> (x/y=w183:dbl)
            n101 = Divide(x=w187, y=w183) -> (x/y=w179:dbl)
            "% Difference" <- w179
            n102 = Select(t="Lo C.- Hi P.", s=w194, f="Z.M.R.") -> (s? t:f=w191:string)
            n103 = Select(t=u32 65336, s=w194, f=u32 16755266) -> (s? t:f=w190:u32)
            n104 = Absolute Value(x=w179) -> (abs(x)=w176:dbl)
            n105 = Less?(x=w176, y="percent warning") -> (x < y?=w177:bool)
            n106 = Select(t=u32 65343, s=w177, f=u32 15668992) -> (s? t:f=w175:u32)
            n107 = property on="zmr 2" class="DigNum (strict)"("Caption.Text"=w191, "Numeric Text.Text Colors:BG Color"=w190) -> ()  [unwired: 2 in, 2 out]
            n108 = property on="% Difference" class="DigNum (strict)"("Numeric Text.Text Colors:BG Color"=w175) -> ()  [unwired: 2 in, 2 out]
            "BACKFACE DIAMETER" <- "backfacedia"
            "BACKFACE DEPTH" <- "backdepth"
          }
          frame #2 {
            n109 = local read "Distance Units"() -> (w219:string)
            n110 = local read "red/speed"() -> (w218:dbl)
            n111 = local read "factor array"() -> (w231:dbl[])
            n112 = Index Array(array=w231, index="Threat 2") -> (element=w213:dbl)
            "correction coefficient" <- w213
            n113 = call "Velocity Correction.vi"("raw impact"="Current/impact/speed", "distance units"=w219, "raw redundant"=w218, "raw residual"="Current/residual/speed", "screen set midpt to target"="Impac/Target Dist", "residual screen to target"="Residual/Target Dist", "correction coefficient"=w213) -> ("corrected impact"=w214:sgl, "corrected redundant"=→"Corrected Redundant":sgl, "corrected residual"=w209:sgl, "impact factor"=w210:sgl, "conversion factor"=→"metric conversion":sgl, "residual factor"=w211:sgl)  [unwired: 3 in]
            "Residual" <- w211
            "Impact" <- w210
            "Corrected Impact" <- w214
            "Corrected Residual" <- w209
            n114 = Not Equal?(x="Drag Corrected", y="old drag") -> (x != y?=w223:bool)
            n115 = Select(t=w209, s="Drag Corrected", f="Current/residual/speed") -> (s? t:f=→"residual/speed":dbl)
            n116 = Select(t=w214, s="Drag Corrected", f="Current/impact/speed") -> (s? t:f=→"Impact/speed":dbl)
            n117 = Not Equal?(x="Threat 2", y="old threat") -> (x != y?=w224:bool)
            n118 = Or(x=w224, y=w223) -> (x .or. y?=w222:bool)
            n119 = case shown="False" w222 {
              tunnel: "Threat 2" -> [_ w246]
              tunnel: w227 -> [w233 w245]
              tunnel: w211 -> [_ w244]
              tunnel: w210 -> [_ w243]
              tunnel: "Drag Corrected" -> [_ w242]
              tunnel: [w233 w241] -> w221
              frame False {
              }
              frame True {
                n120 = local write "old drag"(w242) -> ()
                n121 = local write "old threat"(w246) -> ()
                n122 = for {
                  tunnel: w245 -> [w249] mode=indexing
                  tunnel: w244 -> [w257]
                  tunnel: w243 -> [w256]
                  tunnel: w242 -> [w253]
                  tunnel: [w251] -> w241 mode=indexing
                  n123 = Unbundle By Name(w249) -> ("Uncorrected Residual"=w250:dbl)
                  n124 = Unbundle By Name(w249) -> ("Uncorrected Impact"=w255:dbl)
                  n125 = Multiply(x=w255, y=w256) -> (x*y=w248:dbl)
                  n126 = Select(t=w248, s=w253, f=w255) -> (s? t:f=w252:dbl)
                  n127 = Multiply(x=w250, y=w257) -> (x*y=w254:dbl)
                  n128 = Select(t=w254, s=w253, f=w250) -> (s? t:f=w247:dbl)
                  n129 = Bundle By Name(cluster=w249, "Corrected Impact"=w248, "IMPACT VELOCITY"=w252, "Corrected residual"=w254, "RESIDUAL  VELOCITY"=w247) -> (w251:T11)
                }
                n130 = property on="Threat 2" class="Ring (strict)"() -> ("Strings []"=w240:string[], "Value"=w239:u32)  [unwired: 2 in, 2 out]
                n131 = Index Array(array=w240, index=w239) -> (element=w238:string)
                n132 = Scan From String(format string="%f " ("Format String"), input string=w238) -> (output 1=w236:dbl)  [unwired: 3 in, 3 out]
                n133 = Multiply(x=0.06479891, y=w236) -> (x*y=w234:dbl)
                n134 = local write "Projectile Mass"(w234) -> ()
              }
            }
            "SHOT STATUS" <- "Current/sthotstatus"
          }
          frame #3 {
            # "> SHOTS >"
            n135 = local read "Layers"() -> (w261:T5)
            n136 = Array Size(array=w261) -> (size(s)=w260:i32)
            n137 = Array Size(array=w258) -> (size(s)=w267:i32)
            n138 = Equal To 0?(x=w260) -> (x = 0?=w266:bool)
            n139 = Equal To 0?(x=w267) -> (x = 0?=w265:bool)
            n140 = Or(x=w266, y=w265) -> (x .or. y?=w264:bool)
            n141 = Select(t=u8 2, s=w264, f=u8 0) -> (s? t:f=w259:u8)
            n142 = property on="Save" class="Bool"("Disabled"=w259) -> ()  [unwired: 2 in, 2 out]
            n143 = property on="String" class="Str"("Visible"=w266) -> ()  [unwired: 2 in, 2 out]
          }
          frame #4 {
            n144 = Array Size(array=w269) -> (size(s)=w268:i32)
            n145 = case shown="1, Default" w268 {
              tunnel: w269 -> [_ w272]
              frame 0 {
              }
              frame 1, Default {
                w270 = dbl[] [] ("Partial")
                # "This section calculates the V50"
                n146 = for {
                  tunnel: [w287] -> w281
                  shift-right: [w287] -> _
                  shift-left: w270 -> [w288]
                  shift-right: [w285] -> _
                  shift-left: w270 -> [w286]
                  tunnel: [w285] -> w282
                  tunnel: w272 -> [w284] mode=indexing
                  n147 = Unbundle By Name(w284) -> ("IMPACT VELOCITY"=w289:dbl, "SHOT STATUS"=w283:u16)
                  n148 = case shown="0, Default" w283 {
                    tunnel: w289 -> [w290 w294]
                    tunnel: [w293 w295] -> w287
                    tunnel: w288 -> [w292 w295]
                    tunnel: w286 -> [w291 w297]
                    tunnel: [w291 w296] -> w285
                    frame 0, Default {
                      n149 = Build Array (concatenate)(w292, w290) -> (w293:dbl[])
                    }
                    frame 1 {
                      n150 = Build Array (concatenate)(w297, w294) -> (w296:dbl[])
                    }
                  }
                }
                n151 = Sort 1D Array(array=w281) -> (sorted array=w280:dbl[])
                n152 = Sort 1D Array(array=w282) -> (sorted array=w273:dbl[])
                n153 = Reverse 1D Array(array=w280) -> (reversed array=w276:dbl[])
                n154 = local read "Maximum Deviation"() -> (w279:dbl)
                n155 = call "Compute V50.vi"("Maximum Deviation"=w279, "Partial"=w276, "Complete"=w273) -> ("zmr"=→"Z.M.R.":sgl, "Points"=w277:i16, "V50"=w271:sgl)
                n156 = Array Size(array=w276) -> (size(s)=→"number of partials":i32)
                n157 = Array Size(array=w273) -> (size(s)=→"number of completes":i32)
                n158 = local write "Complete"(w273) -> ()
                n159 = local write "Value"(w271) -> ()
                n160 = local write "Pairs"(w277) -> ()
                n161 = local write "Partial"(w276) -> ()
              }
            }
          }
          frame #5 {
            n162 = local read "Layers"() -> (w300:T5)
            n163 = for {
              tunnel: w300 -> [w308] mode=indexing
              shift-right: [w305] -> w299
              shift-left: u16 0 -> [w306]
              n164 = Unbundle By Name(w308) -> ("Number of Plies"=w307:i32)
              n165 = Greater Than 0?(x=w307) -> (x > 0?=w304:bool)
              n166 = Select(t=u16 1 ("y"), s=w304, f=u16 0) -> (s? t:f=w301:u16)
              n167 = Add(x=w306, y=w301) -> (x+y=w305:u16)
            }
            "plytypes" <- w299
          }
          frame #6 {
            # "This section plots  Impact velocity vs. loadingdata"
            n168 = Not(x="velocity-loading") -> (.not. x?=w315:bool)
            n169 = case shown="False" w315 {
              tunnel: "Powder" -> [w341 _]
              tunnel: "Earliest Date" -> [w344 _]
              tunnel: "Threat" -> [w342 _]
              tunnel: "latest Date" -> [w338 _]
              tunnel: w309 -> [w324 _]
              frame False {
                w320 = FALSE ("Visible")
                w321 = TRUE ("Visible")
                w345 = "" ("replace string (\"\")")
                n170 = invoke on="v50 data 2" class="Tbl" method="Reinit To Default"() -> (error out=w343:errorcluster)  [unwired: 3 in, 2 out]
                n171 = call "Trim String.vi"("inStr"=w342) -> ("outStr"=w340:string)
                n172 = call "Trim String.vi"("inStr"=w341) -> ("outStr"=w339:string)
                n173 = invoke on="Velocity  versus Loading" class="XYGraph (strict)" method="Reinit To Default"(error in=w343) -> (error out=w317:errorcluster)  [unwired: 2 in, 2 out]
                n174 = property on="Data retrieval" class="Str"(error in=w317, "Visible"=w321, "Blinking"=w321) -> (error out=w316:errorcluster)  [unwired: 1 in, 1 out]
                n175 = Format Into String(format string="  select top %d experiment.threat,  shots.loading, shots.impact,  experiment.powder, shots.date from shots, experiment where shots.expt = experiment.expt and shots.loading > .02 and shots.date between  #%s# and #%s# and shots.impact between 5000 and 10 and experiment.powder like '%%%s%%' and experiment.threat like '%%%s%%' and experiment.threat<>'' order by experiment.threat, shots.loading,shots.impact" ("Format String"), error in=w316, "?", w344, w338, w339, w340) -> (resulting string=w349:string, error out=w318:errorcluster)  [unwired: 1 in]
                n176 = call-poly <vilib>:"DB Tools Open Connection.vi"("error in (no error)"=w318, "connection information"=w324) -> ("error out"=w330:errorcluster, "connection reference"=w332:T12)  [unwired: 6 in]
                n177 = Search and Replace String(input string=w349, search string=" and experiment.powder like '%%'", replace string=w345) -> (result string=w347:string)  [unwired: 5 in, 3 out]
                n178 = Search and Replace String(input string=w347, search string="and experiment.threat like '%%'", replace string=w345) -> (result string=w325:string)  [unwired: 5 in, 3 out]
                n179 = call-poly <vilib>:"DB Tools Execute Query.vi"("error in (no error)"=w330, "SQL query"=w325, "connection reference"=w332) -> ("error out"=w329:errorcluster, "recordset reference"=w333:T13)  [unwired: 5 in]
                n180 = call <vilib>:"DB Tools Fetch Table Data.vi"("error in (no error)"=w329, "recordset reference"=w333) -> ("error out"=w328:errorcluster, "recordset data"=w326:string[][], "recordset reference out"=w334:T13)  [unwired: 3 in]
                "v50 data 2" <- w326
                n181 = call-poly <vilib>:"DB Tools Free Object.vi"("error in (no error)"=w328, "recordset reference"=w334) -> ("error out"=w327:errorcluster, "connection reference"=w331:T12)  [unwired: 8 in]
                n182 = call <vilib>:"DB Tools Close Connection.vi"("error in (no error)"=w327, "connection reference"=w331) -> ("error out"=w323:errorcluster)  [unwired: 5 in]
                n183 = Array Size(array=w326) -> (size(s)=w336:i32[])
                n184 = Fract/Exp String To Number(string=w326) -> (number=w353:dbl[][])  [unwired: 3 in, 1 out]
                n185 = call "Continue DB Error Dialog.vi"("error in (no error)"=w323) -> ("error out"=w319:errorcluster)  [unwired: 3 in, 2 out]
                n186 = Index Array(array=w336) -> (element=→"Actual Number of \nRecords Returned":i32)  [unwired: 1 in]
                n187 = Index Array(array=w353, index (col)=2 ("Disabled Index (col)")) -> (element=w352:dbl[])  [unwired: 1 in]
                n188 = Index Array(array=w353, index (col)=1 ("Disabled Index (col)")) -> (element=w351:dbl[])  [unwired: 1 in]
                n189 = Bundle(w351, w352) -> (→"Velocity  versus Loading":cluster{dbl[], dbl[]})  [unwired: 1 in]
                n190 = property on="Data retrieval" class="Str"(error in=w319, "Visible"=w320, "Blinking"=w320) -> ()  [unwired: 1 in, 2 out]
              }
              frame True {
              }
            }
          }
          frame #7 {
            # "This section plots panel V50 data"
            n191 = Not(x="Panel Search") -> (.not. x?=w357:bool)
            n192 = case shown="False" w357 {
              tunnel: w356 -> [w364 _]
              frame False {
                n193 = invoke on="v50 data" class="Tbl" method="Reinit To Default"() -> (error out=w401:errorcluster)  [unwired: 3 in, 2 out]
                n194 = property on="Threat" class="Ring (strict)"() -> ("Strings []"=w399:string[], "Value"=w400:u16)  [unwired: 2 in, 2 out]
                n195 = invoke on="Previous V50 Data" class="WFGraph (strict)" method="Reinit To Default"(error in=w401) -> (error out=w402:errorcluster)  [unwired: 2 in, 2 out]
                n196 = Index Array(array=w399, index=w400) -> (element=w395:string)
                n197 = Format Into String(format string="SELECT  Experiment.Date, Shots.impact\nFROM Shots, Experiment where Shots.Expt = Experiment.expt\nand Experiment.Date Between #%s# And #%s# AND Experiment.threat Like '%%%s%%'\nORDER BY Experiment.Date" ("SQL statement"), error in=w402, "DATE 2", "DATE 3", w395) -> (resulting string=w365:string)  [unwired: 1 in, 1 out]
                n198 = call-poly <vilib>:"DB Tools Open Connection.vi"("connection information"=w364) -> ("error out"=w370:errorcluster, "connection reference"=w372:T12)  [unwired: 7 in]
                n199 = call-poly <vilib>:"DB Tools Execute Query.vi"("error in (no error)"=w370, "SQL query"=w365, "connection reference"=w372) -> ("error out"=w369:errorcluster, "recordset reference"=w373:T13)  [unwired: 5 in]
                n200 = call <vilib>:"DB Tools Fetch Table Data.vi"("error in (no error)"=w369, "recordset reference"=w373) -> ("error out"=w368:errorcluster, "recordset data"=w363:string[][], "recordset reference out"=w374:T13)  [unwired: 3 in]
                n201 = Array Size(array=w363) -> (size(s)=w394:i32[])
                n202 = Index Array(array=w394, index=0 ("Index")) -> (element=w392:i32)
                n203 = call-poly <vilib>:"DB Tools Free Object.vi"("error in (no error)"=w368, "recordset reference"=w374) -> ("error out"=w367:errorcluster, "connection reference"=w371:T12)  [unwired: 8 in]
                n204 = Decrement(x=w392) -> (x-1=w391:i32)
                n205 = call <vilib>:"DB Tools Close Connection.vi"("error in (no error)"=w367, "connection reference"=w371) -> ("error out"=w366:errorcluster)  [unwired: 5 in]
                n206 = Index Array(array=w363, index (row)=w391, index (col)=1 ("Disabled Index (col)")) -> (element=w390:string)
                n207 = Fract/Exp String To Number(string=w390) -> (number=w389:dbl)  [unwired: 3 in, 1 out]
                "Latest Velocity" <- w389
                n208 = call "Continue DB Error Dialog.vi"("error in (no error)"=w366) -> ()  [unwired: 3 in, 3 out]
                n209 = Not Equal?(x=w390, y="") -> (x != y?=w403:bool)
                n210 = Select(t=w363, s=w403, f=string[][] [["", "NONE"], ["", ""]]) -> (s? t:f=→"v50 data":string[][])
                n211 = Fract/Exp String To Number(string=w363) -> (number=w413:dbl[][])  [unwired: 3 in, 1 out]
                n212 = Index Array(array=w413, index (col)=1 ("Disabled Index (col)")) -> (element=w359:dbl[])  [unwired: 1 in]
                n213 = call <vilib>:"Std Deviation and Variance.vi"("X"=w359, "Weighting (Sample)"=enum16{"Sample", "Population"}."Sample") -> ("mean"=w361:dbl, "standard deviation"=w360:dbl)  [unwired: 1 out]
                "Average Velocity" <- w361
                "St. Deviation" <- w360
                n214 = Array Size(array=w359) -> (size(s)=w382:i32)
                n215 = Subtract(x=w361, y=w389) -> (x-y=w388:dbl)
                n216 = Absolute Value(x=w388) -> (abs(x)=w387:dbl)
                n217 = Multiply(x=3.0, y=w360) -> (x*y=w383:dbl)
                n218 = Divide(x=w387, y=w360) -> (x/y=w376:dbl)
                n219 = Subtract(x=w361, y=w383) -> (x-y=w380:dbl)
                n220 = Add(x=w361, y=w383) -> (x+y=w381:dbl)
                n221 = Initialize Array(w361, w382) -> (w412:dbl[])
                n222 = Format Into String(format string="%3.1f" ("Format String"), w376) -> (resulting string=w377:string)  [unwired: 2 in, 1 out]
                n223 = Initialize Array(w380, w382) -> (w379:dbl[])
                n224 = Initialize Array(w381, w382) -> (w378:dbl[])
                n225 = property on="In Control" class="Bool (strict)"("Boolean Text.Text"=w377) -> ()  [unwired: 2 in, 2 out]
                n226 = Build Array(w359, w412, w379, w378) -> (w409:dbl[][])
                n227 = Greater?(x=3.0, y=w376) -> (0:→"In Control":bool)
                n228 = Bundle(0.0, 1.0, w409) -> (→"Previous V50 Data":cluster{dbl, dbl, dbl[][]})  [unwired: 1 in]
              }
              frame True {
              }
            }
          }
          frame #8 {
            n229 = Sort 1D Array(array=w424) -> (sorted array=w425:T1)
            n230 = local read "Pairs"() -> (w421:i16)
            n231 = for {
              tunnel: w425 -> [w483] mode=indexing
              tunnel: [w484] -> w419 mode=indexing
              tunnel: w421 -> [w471]
              shift-right: [w470] -> _
              shift-left: 0 -> [w469]
              # "this section marks the lowest completes that are used in V50"
              n232 = Unbundle By Name(w483) -> ("SHOT STATUS"=w467:u16, "IMPACT VELOCITY"=w475:dbl, "RESIDUAL  VELOCITY"=w474:dbl, "Projectile Mass"=w473:dbl)
              n233 = local read "metric conversion"() -> (w476:dbl)
              n234 = Multiply(x=w476, y=w474) -> (x*y=w477:dbl)
              n235 = Multiply(x=w475, y=w476) -> (x*y=w478:dbl)
              n236 = case shown="0, Default" w467 {
                tunnel: w471 -> [_ w491]
                tunnel: [FALSE w490] -> w468
                tunnel: [w486 w489] -> w470
                tunnel: w469 -> [w486 w487]
                frame 0, Default {
                }
                frame 1 {
                  n237 = Less?(x=w487, y=w491) -> (x < y?=w490:bool)
                  n238 = Add(x=w487, y=1 ("t")) -> (x+y=w489:i32)
                }
              }
              n239 = Multiply(x=w478, y=w478) -> (x*y=w482:dbl)
              n240 = Multiply(x=w477, y=w477) -> (x*y=w481:dbl)
              n241 = Subtract(x=w482, y=w481) -> (x-y=w480:dbl)
              n242 = Compound Arithmetic op=MULTIPLY(w473, w480, 0.0005 ("Input")) -> (w472:dbl)
              n243 = Bundle By Name(cluster=w483, "usedv50"=w468, "Energy Loss (J)"=w472) -> (w484:T11)
            }
            n244 = Reverse 1D Array(array=w419) -> (reversed array=w418:T1)
            n245 = for {
              tunnel: w418 -> [w447] mode=indexing
              tunnel: w421 -> [w450]
              shift-right: [w448] -> _
              shift-left: i16 0 -> [w449]
              tunnel: [w445] -> w420 mode=indexing
              # "chooses highest partials used in v50"
              n246 = Unbundle By Name(w447) -> ("SHOT STATUS"=w451:u16, "usedv50"=w444:bool)
              n247 = case shown="0, Default" w451 {
                tunnel: w450 -> [w455 _]
                tunnel: [w454 w458] -> w446
                tunnel: w449 -> [w452 w457]
                tunnel: [w453 w457] -> w448
                tunnel: w444 -> [_ w458]
                frame 0, Default {
                  n248 = Less?(x=w452, y=w455) -> (x < y?=w454:bool)
                  n249 = Add(x=w452, y=i16 1) -> (x+y=w453:i16)
                }
                frame 1 {
                }
              }
              n250 = Bundle By Name(cluster=w447, "usedv50"=w446) -> (w445:T11)
            }
            n251 = Not Equal?(x=w420, y="old shots") -> (x != y?=w426:bool)
            n252 = case shown="True" w426 {
              tunnel: w420 -> [_ w492]
              frame False {
              }
              frame True {
                n253 = call "Sort Shots.vi"("shot array"=w492) -> ("shotTable OUT"=w493:string[][])
                n254 = local write "old shots"(w492) -> ()
                n255 = local write "SHOTS"(w492) -> ()
                n256 = local write "Table of Shots"(w493) -> ()
              }
            }
            n257 = case shown="True" "Next Shot" {
              tunnel: w420 -> [_ w460]
              frame False {
              }
              frame True {
                n258 = property on="SHOTS" class="Arr (strict)"() -> ("Index Values"=w459:u32[])  [unwired: 2 in, 2 out]
                n259 = Index Array(array=w459) -> (element=w465:u32)  [unwired: 1 in]
                n260 = Array Size(array=w460) -> (size(s)=w463:i32)
                n261 = Increment(x=w465) -> (x+1=w464:u32)
                n262 = Quotient & Remainder(x=w464, y=w463) -> (x-y*floor(x/y)=w462:u32)  [unwired: 1 out]
                n263 = Replace Array Subset(array=w459, new element=w462) -> (w461:u32[])  [unwired: 1 in]
                n264 = local write "Next Shot"(FALSE ("Boolean")) -> ()
                n265 = property on="SHOTS" class="Arr (strict)"("Index Values"=w461) -> ()  [unwired: 2 in, 2 out]
              }
            }
            n266 = case shown="True" "Stop Program" {
              frame False {
              }
              frame True {
                n267 = Stop() -> ()  [unwired: 1 in]
              }
            }
            n268 = Or(x="RESET", y="reread") -> (x .or. y?=w442:bool)
            n269 = Or(x="Reject shot", y="Delete Button") -> (x .or. y?=w437:bool)
            n270 = Build Array("EXIT", w442, "Report", "Save", "switch", "Accept Data", "RANGE RESET", w437, "Contact Shot Report") -> (w430:bool[])
            n271 = Search 1D Array(1D array=w430, element=TRUE) -> (index of element=w429:i32)  [unwired: 1 in]
          }
        }
      }
      frame 0 {
        w495 = -1 ("index of element")
        # "This section stops program"
        n272 = Two Button Dialog(message="All Unsaved data will be lost.   Do you want to quit the program? ") -> (T button?=w497:bool)  [unwired: 2 in]
        n273 = case shown="True" w497 {
          frame False {
          }
          frame True {
            n274 = Quit LabVIEW(quit? (T)=TRUE) -> ()
          }
        }
      }
      frame 1 {
        # "This section reads the ini file"
        # "This section resets the entire program"
        n275 = case shown="100" w503 {
          tunnel: [w506 TRUE] -> w504
          frame 0, Default {
            n276 = local read "RESET"() -> (w505:bool)
            n277 = case shown="True" w505 {
              tunnel: [TRUE w508] -> w506
              frame False {
              }
              frame True {
                n278 = Two Button Dialog(message="Reset will remove all unsaved data.  Do you want to RESET? ") -> (T button?=w508:bool)  [unwired: 2 in]
              }
            }
          }
          frame 100 {
          }
        }
        n279 = case shown="True" w504 {
          tunnel: w502 -> [_ w514]
          tunnel: w501 -> [_ w513]
          tunnel: [-1 ("index of element") w512] -> w500
          frame False {
          }
          frame True {
            n280 = stacked-sequence {
              tunnel: w514 -> [_ w519 _]
              tunnel: w513 -> [_ w521 _]
              tunnel: [_ w517 _] -> w512
              frame #0 {
                n281 = case shown="True" "Case Constant 1" {
                  frame False {
                  }
                  frame True {
                    w516 = TRUE ("Visible")
                    n282 = property on="String 2" class="Str"("Visible"=w516, "Blinking"=w516) -> ()  [unwired: 2 in, 2 out]
                  }
                }
              }
              frame #1 {
                n283 = property on="Method" class="Ring (strict)"() -> ("Label.Text"=w536:string)  [unwired: 2 in, 2 out]
                n284 = property on="ballistician" class="Ring (strict)"() -> ("Label.Text"=w551:string)  [unwired: 2 in, 2 out]
                n285 = property on="Type" class="Ring (strict)"() -> ("Label.Text"=w553:string)  [unwired: 2 in, 2 out]
                n286 = property on="Panel Technician" class="Ring (strict)"() -> ("Label.Text"=w554:string)  [unwired: 2 in, 2 out]
                n287 = property on="Manufacturer" class="Ring (strict)"() -> ("Label.Text"=w562:string)  [unwired: 2 in, 2 out]
                n288 = property on="Type" class="Ring (strict)"() -> ("Label.Text"=w538:string)  [unwired: 2 in, 2 out]
                n289 = property on="Test Conditions" class="Ring (strict)"() -> ("Label.Text"=w561:string)  [unwired: 2 in, 2 out]
                n290 = property on="Panel Backing" class="Ring (strict)"() -> ("Label.Text"=w550:string)  [unwired: 2 in, 2 out]
                n291 = property on="Submitter" class="Ring (strict)"() -> ("Label.Text"=w546:string)  [unwired: 2 in, 2 out]
                n292 = property on="Panel Dimensions" class="Ring (strict)"() -> ("Label.Text"=w548:string)  [unwired: 2 in, 2 out]
                n293 = property on="Powder Type" class="Ring (strict)"() -> ("Label.Text"=w556:string)  [unwired: 2 in, 2 out]
                n294 = property on="Panel Type" class="Ring (strict)"() -> ("Label.Text"=w559:string)  [unwired: 2 in, 2 out]
                n295 = property on="Panel Stitch" class="Ring (strict)"() -> ("Label.Text"=w540:string)  [unwired: 2 in, 2 out]
                n296 = call "Read INI Section 2.vi"("section"=w551, "configuration file path"=w519) -> ("Array"=w552:string[])  [unwired: 4 in, 1 out]
                n297 = call "Read INI Section 2.vi"("section"=w553, "configuration file path"=w519) -> ("Array"=w537:string[])  [unwired: 4 in, 1 out]
                n298 = call "Read INI Section 2.vi"("section"=w554, "configuration file path"=w519) -> ("Array"=w555:string[])  [unwired: 4 in, 1 out]
                n299 = call "Read INI Section 2.vi"("section"=w562, "configuration file path"=w519) -> ("Array"=w557:string[])  [unwired: 4 in, 1 out]
                n300 = call "Read INI Section 2.vi"("section"=w538, "configuration file path"=w519) -> ("Array"=w543:string[])  [unwired: 4 in, 1 out]
                n301 = call "Read INI Section 2.vi"("section"=w561, "configuration file path"=w519) -> ("Array"=w560:string[])  [unwired: 4 in, 1 out]
                n302 = call "Read INI Section 2.vi"("section"=w550, "configuration file path"=w519) -> ("Array"=w549:string[])  [unwired: 4 in, 1 out]
                n303 = call "Read INI Section 2.vi"("section"=w546, "configuration file path"=w519) -> ("Array"=w545:string[])  [unwired: 4 in, 1 out]
                n304 = call "Read INI Section 2.vi"("section"=w548, "configuration file path"=w519) -> ("Array"=w547:string[])  [unwired: 4 in, 1 out]
                n305 = call "Read INI Section 2.vi"("section"=w556, "configuration file path"=w519) -> ("Array"=w544:string[])  [unwired: 4 in, 1 out]
                n306 = call "Read INI Section 2.vi"("section"=w559, "configuration file path"=w519) -> ("Array"=w558:string[])  [unwired: 4 in, 1 out]
                n307 = call "Read INI Section 2.vi"("section"=w540, "configuration file path"=w519) -> ("Array"=w539:string[])  [unwired: 4 in, 1 out]
                n308 = call "Read INI Section 2.vi"("section"="Threat with Correction Factor", "configuration file path"=w519) -> ("Array"=w533:string[])  [unwired: 4 in, 1 out]
                n309 = call "Read INI Section 2.vi"("section"=w536, "configuration file path"=w519) -> ("Array"=w535:string[])  [unwired: 4 in, 1 out]
                n310 = call "Read Parameters.vi"("appended path"=w519) -> ("max dev"=w527:dbl, "barrel screen dist"=w522:dbl, "residual separation"=w526:dbl, "impact separation"=w525:dbl, "impact target dist"=w524:dbl, "resid target dist"=w523:dbl)
                n311 = local write "Maximum Deviation"(w527) -> ()
                n312 = local write "Residual/Separation"(w526) -> ()
                n313 = local write "Impact/Separation"(w525) -> ()
                n314 = local write "Barrel to Screen Distance"(w522) -> ()
                n315 = property on="Method" class="Ring (strict)"("Strings []"=w535) -> ()  [unwired: 2 in, 2 out]
                n316 = local write "Residual/Target Dist"(w523) -> ()
                n317 = property on="ballistician" class="Ring (strict)"("Strings []"=w552) -> ()  [unwired: 2 in, 2 out]
                n318 = property on="Type" class="Ring (strict)"("Strings []"=w537) -> ()  [unwired: 2 in, 2 out]
                n319 = property on="Ply Description" class="Ring (strict)"("Strings []"=w537) -> ()  [unwired: 2 in, 2 out]
                n320 = property on="Panel Technician" class="Ring (strict)"("Strings []"=w555) -> ()  [unwired: 2 in, 2 out]
                n321 = property on="Manufacturer" class="Ring (strict)"("Strings []"=w557) -> ()  [unwired: 2 in, 2 out]
                n322 = property on="Test Conditions" class="Ring (strict)"("Strings []"=w560) -> ()  [unwired: 2 in, 2 out]
                n323 = property on="Panel Backing" class="Ring (strict)"("Strings []"=w549) -> ()  [unwired: 2 in, 2 out]
                n324 = property on="Submitter" class="Ring (strict)"("Strings []"=w545) -> ()  [unwired: 2 in, 2 out]
                n325 = property on="Panel Dimensions" class="Ring (strict)"("Strings []"=w547) -> ()  [unwired: 2 in, 2 out]
                n326 = property on="Powder Type" class="Ring (strict)"("Strings []"=w544) -> ()  [unwired: 2 in, 2 out]
                n327 = property on="Panel Type" class="Ring (strict)"("Strings []"=w558) -> ()  [unwired: 2 in, 2 out]
                n328 = property on="Panel Stitch" class="Ring (strict)"("Strings []"=w539) -> ()  [unwired: 2 in, 2 out]
                n329 = local write "Impac/Target Dist"(w524) -> ()
                n330 = call "Split Factor Array.vi"("Split character"=":", "STRING INPUT"=w533) -> ("FACTOR OUTPUT"=→"factor array":sgl[], "STRING OUTPUT"=w531:string[])
                n331 = property on="Projectile" class="Ring (strict)"("Strings []"=w531) -> ()  [unwired: 2 in, 2 out]
                n332 = property on="Threat 2" class="Ring (strict)"("Strings []"=w531) -> ()  [unwired: 2 in, 2 out]
                n333 = Insert Into Array(array=w543, index=0 ("Index"), new element="ANY STYLE" ("New Element/Subarray")) -> ()  [unwired: 1 out]
                n334 = local read "RESET"() -> (w520:bool)
                n335 = case shown="True" w520 {
                  tunnel: w519 -> [_ _]
                  tunnel: w521 -> [_ w600]
                  tunnel: [errorcluster {"status"=FALSE, "code"=0, "source"=""} ("error out") w575] -> w518
                  frame False {
                  }
                  frame True {
                    w574 = 0  # i32
                    w583 = 0 ("index (row)")
                    w577 = 0 ("index")
                    n336 = call-poly <vilib>:"DB Tools Open Connection.vi"("prompt? (F)"=FALSE ("prompt? (f)"), "connection information"=w600) -> ("error out"=w580:errorcluster, "connection reference"=w578:T12)  [unwired: 6 in]
                    n337 = call <vilib>:"DB Tools Select Data.vi"("error in (no error)"=w580, "columns"=string[] ["max(expt)"], "table"=" experiment ", "connection reference"=w578) -> ("error out"=w590:errorcluster, "data"=w596:variant[][], "connection reference out"=w594:T12)  [unwired: 2 in]
                    n338 = Index Array(array=w596, index (row)=w583) -> (element=w597:variant[])  [unwired: 1 in]
                    n339 = Index Array(array=w597, index=w583) -> (element=w595:variant)
                    n340 = xnode "Database Variant To Data"("database variant"=w595, "error in (no error)"=w590, "type"=w574) -> ("data"=→"Panel":i32, "error out"=w589:errorcluster)
                    n341 = call <vilib>:"DB Tools Select Data.vi"("error in (no error)"=w589, "columns"=string[] ["max(id)"], "table"="shots", "connection reference"=w594) -> ("error out"=w588:errorcluster, "data"=w586:variant[][], "connection reference out"=w593:T12)  [unwired: 2 in]
                    n342 = Index Array(array=w586, index (row)=w577) -> (element=w585:variant[])  [unwired: 1 in]
                    n343 = Index Array(array=w585, index=w577) -> (element=w584:variant)
                    n344 = xnode "Database Variant To Data"("database variant"=w584, "error in (no error)"=w588, "type"=w574) -> ("data"=→"Shot":i32, "error out"=w587:errorcluster)
                    n345 = call <vilib>:"DB Tools Close Connection.vi"("error in (no error)"=w587, "connection reference"=w593) -> ("error out"=w576:errorcluster)  [unwired: 5 in]
                    n346 = call "Continue DB Error Dialog.vi"("error in (no error)"=w576) -> ("error out"=w575:errorcluster)  [unwired: 3 in, 2 out]
                  }
                }
                n347 = case shown="True" w520 {
                  tunnel: [-1 ("index of element") w564] -> w517
                  frame False {
                  }
                  frame True {
                    n348 = invoke on="Complete" class="Arr (strict)" method="Reinit To Default"() -> ()  [unwired: 3 in, 3 out]
                    n349 = invoke on="Impact/speed" class="DigNum (strict)" method="Reinit To Default"() -> ()  [unwired: 3 in, 3 out]
                    n350 = invoke on="Drag Corrected" class="Bool (strict)" method="Reinit To Default"() -> ()  [unwired: 3 in, 3 out]
                    n351 = invoke on="Value" class="DigNum (strict)" method="Reinit To Default"() -> ()  [unwired: 3 in, 3 out]
                    n352 = local write "RESET"(FALSE) -> ()
                    n353 = invoke on="Partial" class="Arr (strict)" method="Reinit To Default"() -> ()  [unwired: 3 in, 3 out]
                    n354 = invoke on="residual/speed" class="DigNum (strict)" method="Reinit To Default"() -> ()  [unwired: 3 in, 3 out]
                    n355 = invoke on="Pairs" class="DigNum (strict)" method="Reinit To Default"() -> ()  [unwired: 3 in, 3 out]
                    n356 = invoke on="SHOTS" class="Arr (strict)" method="Reinit To Default"() -> (error out=w566:errorcluster)  [unwired: 3 in, 2 out]
                    n357 = invoke on="Shot Decription" class="Str" method="Reinit To Default"() -> ()  [unwired: 3 in, 3 out]
                    n358 = invoke on="Save" class="Bool" method="Reinit To Default"() -> ()  [unwired: 3 in, 3 out]
                    n359 = invoke on="Accept Data" class="Bool (strict)" method="Reinit To Default"() -> ()  [unwired: 3 in, 3 out]
                    n360 = invoke on="Table of Shots" class="Tbl" method="Reinit To Default"(error in=w566) -> ()  [unwired: 2 in, 3 out]
                    n361 = local read "Data Source"() -> (w567:u16)
                    n362 = invoke on="old shots" class="Arr (strict)" method="Reinit To Default"() -> ()  [unwired: 3 in, 3 out]
                    n363 = invoke on="Z.M.R." class="DigNum (strict)" method="Reinit To Default"() -> ()  [unwired: 3 in, 3 out]
                    n364 = invoke on="old threat" class="DigNum (strict)" method="Reinit To Default"() -> ()  [unwired: 3 in, 3 out]
                    n365 = case shown="2" w567 {
                      tunnel: [-1 ("index of element") -1 ("index of element") 6 ("index of element")] -> w564
                      frame 0, Default {
                      }
                      frame 1 {
                      }
                      frame 2 {
                        # "check for PCI 6602"
                      }
                    }
                    n366 = invoke on="old drag" class="Bool (strict)" method="Reinit To Default"() -> ()  [unwired: 3 in, 3 out]
                  }
                }
                n367 = Path To String(path=w519) -> (string=w528:string)
                n368 = invoke on="Stop Program" class="Bool (strict)" method="Reinit To Default"() -> ()  [unwired: 3 in, 3 out]
                n369 = case shown="False" "message control" {
                  tunnel: w518 -> [_ _]
                  tunnel: w528 -> [w571 _]
                  frame False {
                    n370 = call "Ballistics Message Center.vi"("INI File Name"=w571) -> ()
                    n371 = local write "message control"(TRUE) -> ()
                  }
                  frame True {
                  }
                }
              }
              frame #2 {
                n372 = stacked-sequence {
                  frame #0 {
                    n373 = property on="String 2" class="Str"("Visible"=FALSE) -> ()  [unwired: 2 in, 2 out]
                  }
                  frame #1 {
                    n374 = One Button Dialog(message="     Ballistic Test Program is now ready for use") -> ()  [unwired: 1 in, 1 out]
                  }
                }
              }
            }
          }
        }
      }
      frame 2 {
        w708 = TRUE  # append on new line? (F)
        w750 = TRUE  # append on new line? (F)
        w786 = FALSE  # show grid lines
        w798 = -1 ("index of element")
        # "This section prepares a V50 report"
        # "add graph to 3rd box"
        n375 = invoke on="Shot Graph" class="XYGraph (strict)" method="Reinit To Default"() -> (error out=w764:errorcluster)  [unwired: 3 in, 2 out]
        n376 = control-ref of="Value"() -> (w762:refnum<vi>)
        n377 = control-ref of="Points"() -> (w760:refnum<vi>)
        n378 = control-ref of="Complete"() -> (w761:refnum<vi>)
        n379 = control-ref of="Partial"() -> (w759:refnum<vi>)
        n380 = call "Graph V50.vi"("valueRef"=w762, "completeRef"=w761, "pointsRef"=w760, "partialRef"=w759, "error IN"=w764) -> ("shotGraph"=→"Shot Graph":cluster{i32[], sgl[]}[])
        n381 = property on="Submitter" class="Ring (strict)"() -> ("Strings []"=w695:string[], "Value"=w694:u16)  [unwired: 2 in, 2 out]
        n382 = local read "Panel"() -> (w690:i32)
        n383 = Index Array(array=w695, index=w694) -> (element=w691:string)
        n384 = call <vilib>:"New Report.vi"("report type"=enum16{"Standard Report", "HTML"}."HTML", "error in (no error)"=w764) -> ("report out"=w788:refnum<class "NI_report.lvclass">, "error out"=w787:errorcluster)  [unwired: 12 in]
        n385 = Format Into String(format string="Serial Number: %5d<newline>Submitter: %s" ("Format String"), w690, w691) -> (resulting string=w689:string)  [unwired: 2 in, 1 out]
        n386 = call-dynamic "Set Report Font.vi"("report in"=w788, "text options"=T10 {"Italic"=enum."Italic Unchanged", "Strike Through"=enum."Strike Through Unchanged", "Underline"=enum."Underline Unchanged", "Bold"=enum."Bold On"}, "font settings"=T9 {"Charset (-1)"=-1, "Weight (-1)"=-1, "Name"="Arial", "Size"="4 "}, "error in (no error)"=w787) -> ("report out"=w771:refnum<class "NI_report.lvclass">, "error out"=w772:errorcluster)  [unwired: 9 in, 1 out]
        n387 = local read "Fabric Description"() -> (w720:string)
        n388 = property on="Threat 2" class="Ring (strict)"() -> ("Strings []"=w719:string[], "Value"=w718:u32)  [unwired: 2 in, 2 out]
        n389 = local read "Areal Density"() -> (w669:dbl)
        n390 = property on="Panel Backing" class="Ring (strict)"() -> ("Strings []"=w725:string[], "Value"=w724:u16)  [unwired: 2 in, 2 out]
        n391 = property on="Powder Type" class="Ring (strict)"() -> ("Strings []"=w723:string[], "Value"=w722:u16)  [unwired: 2 in, 2 out]
        n392 = property on="Manufacturer" class="Ring (strict)"() -> ("Strings []"=w727:string[], "Value"=w726:u32)  [unwired: 2 in, 2 out]
        n393 = Index Array(array=w719, index=w718) -> (element=w676:string)
        n394 = call-dynamic "Set Report Header Text.vi"("report in"=w771, "left header text"=w689, "center header text"="PBBA Ballistic V50 Report ", "error in (no error)"=w772, "HTML header size"=enum16{"H1", "H2", "H3", "H4", "H5", "H6", "H7"}."H1") -> ("report out"=w774:refnum<class "NI_report.lvclass">, "error out"=w775:errorcluster)  [unwired: 9 in]
        n395 = Index Array(array=w725, index=w724) -> (element=w670:string)
        n396 = Index Array(array=w723, index=w722) -> (element=w711:string)
        n397 = Index Array(array=w727, index=w726) -> (element=w721:string)
        n398 = local read "Room Temperature"() -> (w673:i32)
        n399 = local read "Projectile Mass"() -> (w671:dbl)
        n400 = local read "Impact"() -> (w717:dbl)
        n401 = call-dynamic "Set Report Font.vi"("report in"=w774, "text options"=T10 {"Italic"=enum."Italic Unchanged", "Strike Through"=enum."Strike Through Unchanged", "Underline"=enum."Underline Unchanged", "Bold"=enum."Bold Off"}, "font settings"=T9 {"Charset (-1)"=-1, "Weight (-1)"=-1, "Name"="Arial", "Size"="1"}, "error in (no error)"=w775) -> ("report out"=w745:refnum<class "NI_report.lvclass">, "error out"=w746:errorcluster)  [unwired: 9 in, 1 out]
        n402 = Select(t="Disclosure on Ballistic and Stab Test Data<newline>The attached ballistic test data was generated by PBBA and corresponds to PBBA's current knowledge on the performance of the subject test panels against certain ballistic threats.  This information is offered solely to provide possible suggestions for your own experimentation and validation.  It is not intended as a substitute for your own testing or any testing you may need to submit for a bid package, you should undertake your own testing whether you do so yourself with the supplier of the materials to be tested or with an independent, third party, certified testing facility and the supplier of the materials to be tested (i.e., the fabric weaver).  PBBA makes no warranties, and assumes no liabilities in connection with any use of the information supplied with this disclosure statement." ("text"), s="Add Disclaimer", f="" ("t")) -> (s? t:f=w704:string)
        n403 = call-poly <vilib>:"Append Report Text.vi"("report in"=w745, "text"=w704, "error in (no error)"=w746) -> ("report out"=w744:refnum<class "NI_report.lvclass">, "error out"=w742:errorcluster)  [unwired: 9 in, 2 out]
        n404 = call-dynamic "Set Report Font.vi"("report in"=w744, "text options"=T10 {"Italic"=enum."Italic Unchanged", "Strike Through"=enum."Strike Through Unchanged", "Underline"=enum."Underline Unchanged", "Bold"=enum."Bold Unchanged"}, "font settings"=T9 {"Charset (-1)"=-1, "Weight (-1)"=-1, "Name"="Arial", "Size"="3 "}, "error in (no error)"=w742) -> ("report out"=w743:refnum<class "NI_report.lvclass">, "error out"=w741:errorcluster)  [unwired: 9 in, 1 out]
        n405 = local read "Sample ID"() -> (w668:string)
        n406 = local read "Weight of Panel"() -> (w672:dbl)
        n407 = local read "Room Humidity"() -> (w675:i32)
        n408 = property on="Panel Type" class="Ring (strict)"() -> ("Strings []"=w714:string[], "Value"=w713:u32)  [unwired: 2 in, 2 out]
        n409 = property on="Test Conditions" class="Ring (strict)"() -> ("Strings []"=w716:string[], "Value"=w715:u32)  [unwired: 2 in, 2 out]
        n410 = call-dynamic "New Report Line.vi"("report in"=w743, "error in (no error)"=w741) -> ("report out"=w789:refnum<class "NI_report.lvclass">, "error out"=w790:errorcluster)  [unwired: 12 in]
        n411 = local read "Shot Angle"() -> (w710:u16)
        n412 = call-dynamic "New Report Line.vi"("report in"=w789, "error in (no error)"=w790) -> ("report out"=w752:refnum<class "NI_report.lvclass">, "error out"=w751:errorcluster)  [unwired: 12 in]
        n413 = Index Array(array=w716, index=w715) -> (element=w709:string)
        n414 = Index Array(array=w714, index=w713) -> (element=w674:string)
        n415 = local read "Z.M.R."() -> (w702:dbl)
        n416 = Format Into String(format string="<table border=\"0\" cellspacing=\"6\"><tr><td align=\"left\"><b>Fabric Parameters</b></td><td>&nbsp;</td><td>&nbsp;</td><td align=\"left\"><b>Test Parameters</b></td><td>&nbsp;</td></tr><tr><td align=\"right\">Sample ID: </td><td align=\"left\">%s</td><td>&nbsp;</td><td align=\"right\">Method: </td><td align=\"left\">V50</td></tr><tr><td align=\"right\">Areal Density: </td><td align=\"left\">%.3f</td><td>&nbsp;</td><td align=\"right\">Threat: </td><td align=\"left\">%s</td></tr><tr><td align=\"right\">Manufacturer: </td><td align=\"left\">%s</td><td>&nbsp;</td><td align=\"right\">Room Temperature: </td><td align=\"left\">%.0f</td></tr><tr><td align=\"right\">Group Data: </td><td align=\"left\">%s</td><td>&nbsp;</td><td align=\"right\">Correction Factor: </td><td align=\"left\">%0.4f</td></tr><tr><td align=\"right\">Projectile Weight: </td><td align=\"left\">%0.3f</td><td>&nbsp;</td><td align=\"right\">Panel Backing: </td><td align=\"left\">%s</td></tr><tr><td align=\"right\">Powder Type: </td><td align=\"left\">%s</td><td>&nbsp;</td><td align=\"right\">Shot Angle: </td><td align=\"left\">%.0f</td></tr><tr><td align=\"right\">Test Conditions: </td><td align=\"left\">%s</td><td>&nbsp;</td><td align=\"right\">Room Humidity: </td><td align=\"left\">%.0f</td></tr><tr><td align=\"right\">Panel Weight: </td><td align=\"left\">%.4f</td><td>&nbsp;</td><td>&nbsp;</td></tr><tr><td align=\"right\">Descripton: </td><td align=\"left\">%s</td><td>&nbsp;</td><td>&nbsp;</td></tr></table>", w668, w669, w676, w721, w673, w720, w717, w671, w670, w711, w710, w709, w675, w672, w674) -> (resulting string=w706:string)  [unwired: 2 in, 1 out]
        n417 = local read "Table of Shots"() -> (w766:string[][])
        n418 = call-poly <vilib>:"Append Report Text.vi"("report in"=w752, "text"=w706, "append on new line? (F)"=w750, "error in (no error)"=w751) -> ("report out"=w682:refnum<class "NI_report.lvclass">, "error out"=w683:errorcluster)  [unwired: 8 in, 2 out]
        n419 = call-dynamic "New Report Line.vi"("report in"=w682, "error in (no error)"=w683) -> ("report out"=w783:refnum<class "NI_report.lvclass">, "error out"=w784:errorcluster)  [unwired: 12 in]
        n420 = Less Than 0?(x=w702) -> (x < 0?=w703:bool)
        n421 = property on="Table of Shots" class="Tbl (strict)"() -> ("Column Header Strings[]"=w763:string[])  [unwired: 2 in, 2 out]
        n422 = property on="ballistician" class="Ring (strict)"() -> ("Strings []"=w731:string[], "Value"=w730:u16)  [unwired: 2 in, 2 out]
        n423 = call-dynamic "New Report Line.vi"("report in"=w783, "error in (no error)"=w784) -> ("report out"=w782:refnum<class "NI_report.lvclass">, "error out"=w781:errorcluster)  [unwired: 12 in]
        n424 = Select(t="Low Complete-High Partial: ", s=w703, f="Zone of Mixed Results: ") -> (s? t:f=w698:string)
        n425 = local read "Pairs"() -> (w728:i16)
        n426 = Index Array(array=w731, index=w730) -> (element=w729:string)
        n427 = call-poly <vilib>:"Append Table to Report.vi"("report in"=w782, "column width (1)"=1.1, "column headers"=w763, "text data"=w766, "error in (no error)"=w781, "show grid lines"=w786) -> ("report out"=w732:refnum<class "NI_report.lvclass">, "error out"=w736:errorcluster)  [unwired: 6 in, 2 out]
        n428 = local read "Value"() -> (w747:dbl)
        n429 = Concatenate Strings(" V50:  %10.1f<newline>Number of Pairs Used: %d<newline>  ", w698, "%.1f<newline><newline>Ballistician:%s<newline> ") -> (w696:string)
        n430 = call-dynamic "Set Report Font.vi"("report in"=w732, "text options"=T10 {"Italic"=enum."Italic Unchanged", "Strike Through"=enum."Strike Through Unchanged", "Underline"=enum."Underline On", "Bold"=enum."Bold Off"}, "font settings"=T9 {"Charset (-1)"=-1, "Weight (-1)"=-1, "Name"="Arial", "Size"="3 "}, "error in (no error)"=w736) -> ("report out"=w733:refnum<class "NI_report.lvclass">, "error out"=w734:errorcluster)  [unwired: 9 in, 1 out]
        n431 = Format Into String(format string=w696, w747, w728, w702, w729) -> (resulting string=w748:string)  [unwired: 2 in, 1 out]
        n432 = control-ref of="Shot Graph"() -> (w707:refnum<vi>)
        n433 = call-dynamic "New Report Line.vi"("report in"=w733, "error in (no error)"=w734) -> ("report out"=w780:refnum<class "NI_report.lvclass">, "error out"=w779:errorcluster)  [unwired: 12 in]
        n434 = call-poly <vilib>:"Append Report Text.vi"("report in"=w780, "text"=w748, "append on new line? (F)"=w708, "error in (no error)"=w779) -> ("report out"=w680:refnum<class "NI_report.lvclass">, "error out"=w679:errorcluster)  [unwired: 8 in, 2 out]
        n435 = local read "Sample ID"() -> (w693:string)
        n436 = Get Date/Time String(date format (0)=enum16{"short", "long", "abbreviated"}."abbreviated") -> (date string=w738:string)  [unwired: 2 in, 1 out]
        n437 = call-dynamic "Append Control Image to Report.vi"("report in"=w680, "image file type (.jpg)"=enum16{".jpg", ".png"}.".jpg" ("image file type(.png)"), "ctrl reference"=w707, "description"="Graph of Test Results" ("control name"), "error in (no error)"=w679) -> ("report out"=w677:refnum<class "NI_report.lvclass">, "error out"=w678:errorcluster)  [unwired: 7 in, 2 out]
        n438 = Concatenate Strings(w738, "© " ("right footer text"), "  Point Blank Body Armor ") -> (w756:string)
        n439 = Format Value(format string="Panel %s.html  " ("string (\"\")"), value (0)=w693) -> (output string=w755:string)  [unwired: 1 in]
        n440 = call-dynamic "Set Report Footer Text.vi"("report in"=w677, "right footer text"=w756, "error in (no error)"=w678) -> ("report out"=w776:refnum<class "NI_report.lvclass">, "error out"=w777:errorcluster)  [unwired: 11 in]
        n441 = Build Path(base path="Report Path", name or relative path=w755) -> (appended path=w753:path)
        n442 = call-dynamic "Get Report Type.vi"("report in"=w776, "error in (no error)"=w777) -> ("report out"=w794:refnum<class "NI_report.lvclass">, "report type"=w793:T14, "error out"=w797:errorcluster)  [unwired: 11 in]
        n443 = case shown="\"Standard Report\", Default" w793 {
          tunnel: w794 -> [w804 w809]
          tunnel: [w803 w808] -> w795
          tunnel: [w802 w807] -> w796
          tunnel: w797 -> [w801 w806]
          tunnel: w753 -> [w800 w805]
          tunnel: [w800 w805] -> _
          frame "Standard Report", Default {
            n444 = call-dynamic "Print Report.vi"("report in"=w804, "error in (no error)"=w801) -> ("report out"=w803:refnum<class "NI_report.lvclass">, "error out"=w802:errorcluster)  [unwired: 12 in]
          }
          frame "HTML" {
            n445 = call-dynamic "Save Report to File.vi"("report in"=w809, "report file path"=w805, "error in (no error)"=w806) -> ("report out"=w808:refnum<class "NI_report.lvclass">, "error out"=w807:errorcluster)  [unwired: 11 in]
          }
        }
        n446 = call-dynamic "Dispose Report.vi"("report in"=w795, "error in (no error)"=w796) -> ("error out"=w684:errorcluster)  [unwired: 13 in]
        n447 = call <vilib>:"Simple Error Handler.vi"("error in (no error)"=w684) -> ("error out"=w685:errorcluster)  [unwired: 4 in, 4 out]
        n448 = case shown="No Error" w685 {
          frame No Error {
            n449 = One Button Dialog(message="A V50 Report is ready.") -> ()  [unwired: 1 in, 1 out]
          }
          frame Error {
          }
        }
      }
      frame 3 {
        # "This section saves the shots to the data base"
        n450 = stacked-sequence {
          seq-local: [w823 _ _] -> [_ w895 _]
          seq-local: [w824 _ _] -> [_ w874 _]
          seq-local: [_ w849 _] -> [_ _ w934]
          seq-local: [_ w851 _] -> [_ _ w933]
          seq-local: [_ w847 _] -> [_ _ w932]
          seq-local: [w821 _ _] -> [_ w846 _]
          seq-local: [w820 _ _] -> [_ w845 _]
          tunnel: w815 -> [_ _ w935]
          tunnel: [_ _ w927] -> w811
          tunnel: [_ _ w930] -> w814
          tunnel: w812 -> [w819 _ _]
          frame #0 {
            n451 = call-poly <vilib>:"DB Tools Open Connection.vi"("connection information"=w819) -> ("error out"=w820:errorcluster, "connection reference"=w821:T12)  [unwired: 7 in]
            n452 = Array Size(array="Layers") -> (size(s)=w828:i32)
            n453 = Format Into String(format string=" VALUES (%d ", w828) -> (resulting string=w827:string)  [unwired: 2 in, 1 out]
            n454 = for {
              tunnel: "Layers" -> [w843] mode=indexing
              shift-right: [w834] -> w824
              shift-left: w827 -> [w837]
              shift-right: [w830] -> w823
              shift-left: "insert into experiment (plytypes " ("SQL statement") -> [w831]
              i -> [w833]
              n455 = Unbundle By Name(w843) -> ("Number of Plies"=w836:i32, "Layer Comments"=w838:string, "Ply Description"=w840:u16)
              n456 = property on="Ply Description" class="Ring (strict)"() -> ("Strings []"=w841:string[])  [unwired: 2 in, 2 out]
              n457 = Increment(x=w833) -> (x+1=w829:i32)
              n458 = Format Into String(format string=", ply%1dnumber, ply%1dtext", initial string=w831, w829, w829) -> (resulting string=w830:string)  [unwired: 1 in, 1 out]
              n459 = Index Array(array=w841, index=w840) -> (element=w839:string)
              n460 = Concatenate Strings(w838, "   " ("Substring"), w839) -> (w835:string)
              n461 = Format Into String(format string=", %d,  '%s'", initial string=w837, w836, w835) -> (resulting string=w834:string)  [unwired: 1 in, 1 out]
            }
          }
          frame #1 {
            w867 = " " ("Substring")
            n462 = property on="Panel Backing" class="Ring (strict)"() -> ("Strings []"=w917:string[], "Value"=w916:u16)  [unwired: 2 in, 2 out]
            n463 = property on="Manufacturer" class="Ring (strict)"() -> ("Strings []"=w923:string[], "Value"=w920:u32)  [unwired: 2 in, 2 out]
            n464 = property on="Panel Type" class="Ring (strict)"() -> ("Strings []"=w924:string[], "Value"=w921:u32)  [unwired: 2 in, 2 out]
            n465 = property on="Method" class="Ring (strict)"() -> ("Strings []"=w899:string[], "Value"=w898:u16)  [unwired: 2 in, 2 out]
            n466 = Index Array(array=w917, index=w916) -> (element=w884:string)
            n467 = Index Array(array=w924, index=w921) -> (element=w863:string)
            n468 = property on="Panel Stitch" class="Ring (strict)"() -> ("Strings []"=w904:string[], "Value"=w903:u32)  [unwired: 2 in, 2 out]
            n469 = Index Array(array=w923, index=w920) -> (element=w888:string)
            n470 = Index Array(array=w899, index=w898) -> (element=w880:string)
            n471 = local read "Drag Corrected"() -> (w854:bool)
            n472 = property on="Type" class="Ring (strict)"() -> ("Strings []"=w919:string[], "Value"=w918:u16)  [unwired: 2 in, 2 out]
            n473 = property on="Powder Type" class="Ring (strict)"() -> ("Strings []"=w907:string[], "Value"=w906:u16)  [unwired: 2 in, 2 out]
            n474 = local read "Panel"() -> (w848:i32)
            n475 = property on="Panel Dimensions" class="Ring (strict)"() -> ("Strings []"=w915:string[], "Value"=w914:u16)  [unwired: 2 in, 2 out]
            n476 = property on="N.I.J" class="Ring (strict)"() -> ("Strings []"=w897:string[])  [unwired: 2 in, 2 out]
            n477 = local read "Impact"() -> (w856:dbl)
            n478 = Index Array(array=w904, index=w903) -> (element=w861:string)
            n479 = Increment(x=w848) -> (x+1=w847:i32)
            n480 = Index Array(array=w919, index=w918) -> (element=w902:string)
            n481 = Index Array(array=w907, index=w906) -> (element=w886:string)
            n482 = Concatenate Strings(w902, w867, w861, w867, w863, w867, "Fabric Description") -> (w860:string)
            n483 = Index Array(array=w897, index="N.I.J") -> (element=w881:string)
            n484 = local read "Value"() -> (w859:dbl)
            n485 = Index Array(array=w915, index=w914) -> (element=w876:string)
            n486 = Select(t=w856, s=w854, f=1.0) -> (s? t:f=w855:dbl)
            n487 = property on="Panel Technician" class="Ring (strict)"() -> ("Strings []"=w866:string[], "Value"=w865:u16)  [unwired: 2 in, 2 out]
            n488 = property on="Test Conditions" class="Ring (strict)"() -> ("Strings []"=w925:string[], "Value"=w922:u32)  [unwired: 2 in, 2 out]
            n489 = property on="Threat 2" class="Ring (strict)"() -> ("Strings []"=w901:string[], "Value"=w900:u32)  [unwired: 2 in, 2 out]
            n490 = property on="Submitter" class="Ring (strict)"() -> ("Strings []"=w913:string[], "Value"=w912:u16)  [unwired: 2 in, 2 out]
            n491 = Divide(x=w859, y=w855) -> (x/y=w858:dbl)
            n492 = Index Array(array=w925, index=w922) -> (element=w909:string)
            n493 = local read "Total Number of Layers"() -> (w883:i32)
            n494 = Index Array(array=w901, index=w900) -> (element=w890:string)
            n495 = Index Array(array=w866, index=w865) -> (element=w864:string)
            n496 = Index Array(array=w913, index=w912) -> (element=w911:string)
            n497 = local read "CURRENT TIME / DATE"() -> (w905:string)
            n498 = property on="ballistician" class="Ring (strict)"() -> ("Strings []"=w870:string[], "Value"=w868:u16)  [unwired: 2 in, 2 out]
            n499 = local read "Shot Angle"() -> (w910:u16)
            n500 = local read "zmr 2"() -> (w871:dbl)
            n501 = local read "SHOTS"() -> (w908:T1)
            n502 = Index Array(array=w870, index=w868) -> (element=w869:string)
            n503 = Array Size(array=w908) -> (size(s)=w885:i32)
            n504 = Format Into String(format string=", %d, #%s#, '%s', '%s', %d, '%s', '%s', %.4f, '%s', '%s', %.4f, %.1f, %.6f, '%s', %.4f, '%s', %d, '%s', %d, '%s', '%s', %d, '%s', %d, %d, %.2f, '%s', %.1f, '%s', '%s' )" ("Format String"), initial string=w874, w847, w905, w869, w911, w910, w909, w860, "Areal Density", "Areal density text", w890, "Weight of Panel", w859, w858, w888, "Thickness", w886, w885, w884, w883, "Test Comments", w881, "B.F.S (mm)", w880, "Room Temperature", "Room Humidity", "Version", w876, w871, "Sample ID", w864) -> (resulting string=w873:string)  [unwired: 1 in, 1 out]
            n505 = Concatenate Strings(w895, ", expt, [date], operator, submitter, angle, conditions, fabric, density, densitytext, threat, panelweight, v50dc, v50 , maker, thickness, powder, numshots, backing, totalnumberplys, testcomments, nij, bfs, method, temperature, humidity, version, dimensions, zmr, sampleid, panelmaker)" ("Substring"), w873) -> (w853:string)
            n506 = call-poly <vilib>:"DB Tools Execute Query.vi"("error in (no error)"=w845, "SQL query"=w853, "connection reference"=w846) -> ("error out"=w852:errorcluster, "recordset reference"=w850:T13)  [unwired: 5 in]
            n507 = call-poly <vilib>:"DB Tools Free Object.vi"("error in (no error)"=w852, "recordset reference"=w850) -> ("error out"=w851:errorcluster, "connection reference"=w849:T12)  [unwired: 8 in]
          }
          frame #2 {
            n508 = local read "Shot"() -> (w931:i32)
            n509 = Increment(x=w931) -> (x+1=w929:i32)
            n510 = for {
              tunnel: w935 -> [w973] mode=indexing
              tunnel: w934 -> [w938]
              tunnel: w933 -> [w940]
              tunnel: [w936] -> w926
              tunnel: [w937] -> w928
              tunnel: w932 -> [w961]
              tunnel: w929 -> [w945]
              tunnel: [w943] -> w930
              i -> [w943]
              n511 = Unbundle By Name(w973) -> ("IMPACT VELOCITY"=w957:dbl, "RESIDUAL  VELOCITY"=w956:dbl, "Shot Description"=w962:string, "Powder Loading"=w963:dbl, "Barrel Temperature"=w964:dbl, "TIME / DATE"=w965:string, "shot order"=w966:i32, "Shot Angle"=w967:u16, "BackFace\nDepth"=w968:dbl, "BackFace\nDiameter"=w969:dbl, "SHOT STATUS"=w971:u16, "Projectile Mass"=w960:dbl, "usedv50"=w959:bool, "Energy Loss (J)"=w958:sgl, "Red Vel"=w946:dbl)
              n512 = local read "Drag Corrected"() -> (w951:bool)
              n513 = Add(x=w945, y=w943) -> (x+y=w944:i32)
              n514 = local read "Residual"() -> (w953:dbl)
              n515 = local read "Impact"() -> (w948:dbl)
              n516 = Greater Than 0?(x=w971) -> (x > 0?=w970:bool)
              n517 = Select(t=w948, s=w951, f=1.0) -> (s? t:f=w950:dbl)
              n518 = Select(t=w953, s=w951, f=1.0) -> (s? t:f=w952:dbl)
              n519 = Divide(x=w956, y=w952) -> (x/y=w955:dbl)
              n520 = Divide(x=w957, y=w950) -> (x/y=w947:dbl)
              n521 = Format Into String(format string="INSERT INTO shots (impactdc, residualdc, comment, loading, barreltemp, [date], [order], shotangle, bfdepth, bfdiameter, [complete], expt, id, weight,usedv50, loss, residual, impact, redundantdc)  VALUES (%.1f, %.1f, '%s', %.4f, %.1f, #%s#, %d, %d, %.3f, %.3f, %d, %d, %d, %.4f, %d, %.4f, %.1f, %.1f, %.1f)" ("Substring"), w957, w956, w962, w963, w964, w965, w966, w967, w968, w969, w970, w961, w944, w960, w959, w958, w955, w947, w946) -> (resulting string=w939:string)  [unwired: 2 in, 1 out]
              n522 = call-poly <vilib>:"DB Tools Execute Query.vi"("error in (no error)"=w940, "SQL query"=w939, "connection reference"=w938) -> ("error out"=w942:errorcluster, "recordset reference"=w941:T13)  [unwired: 5 in]
              n523 = call-poly <vilib>:"DB Tools Free Object.vi"("error in (no error)"=w942, "recordset reference"=w941) -> ("error out"=w936:errorcluster, "connection reference"=w937:T12)  [unwired: 8 in]
            }
            n524 = call <vilib>:"DB Tools Close Connection.vi"("error in (no error)"=w926, "connection reference"=w928) -> ("error out"=w927:errorcluster)  [unwired: 5 in]
          }
        }
        n525 = Unbundle By Name(w811) -> ("status"=w818:bool)
        n526 = case shown="False" w818 {
          tunnel: [100 w995] -> w816
          tunnel: [1 w995] -> w817
          tunnel: w811 -> [_ w994]
          tunnel: w814 -> [w988 _]
          tunnel: w813 -> [w974 _]
          frame False {
            w977 = "Data Base Parameters" ("section")
            n527 = call <vilib>:"Open Config Data (compatibility).vi"("configuration file path"=w974) -> ("error out"=w981:errorcluster, "refnum"=w980:T8)  [unwired: 8 in, 1 out]
            n528 = local read "Shot"() -> (w989:i32)
            n529 = Increment(x=w989) -> (x+1=w983:i32)
            n530 = Add(x=w983, y=w988) -> (x+y=w984:i32)
            n531 = local write "Shot"(w984) -> ()
            n532 = call-poly <vilib>:"Write Key.vi"("section"=w977, "error in (no error)"=w981, "value"=w984, "key"="Last Shot Saved ", "refnum"=w980) -> ("error out"=w979:errorcluster, "refnum out"=w978:T8)  [unwired: 4 in, 1 out]
            n533 = local read "Panel"() -> (w985:i32)
            n534 = Increment(x=w985) -> (x+1=w982:i32)
            n535 = local write "Panel"(w982) -> ()
            n536 = call-poly <vilib>:"Write Key.vi"("section"=w977, "error in (no error)"=w979, "value"=w982, "key"="Last Panel Saved ", "refnum"=w978) -> ()  [unwired: 4 in, 3 out]
            n537 = call <vilib>:"Close Config Data.vi"("error in (no error)"=w979, "refnum"=w978) -> ("error out"=w975:errorcluster)  [unwired: 8 in, 1 out]
            n538 = case shown="True" "Case Constant 2" {
              tunnel: w975 -> [_ _]
              frame False {
              }
              frame True {
                n539 = One Button Dialog(message="Data Saved") -> ()  [unwired: 1 in, 1 out]
              }
            }
          }
          frame True {
            w995 = -1
            n540 = call <vilib>:"Simple Error Handler.vi"("error in (no error)"=w994) -> ()  [unwired: 4 in, 5 out]
            n541 = One Button Dialog(message="Error saving Data. ") -> ()  [unwired: 1 in, 1 out]
          }
        }
      }
      frame 4 {
        w1008 = -1 ("index of element")
        # "This section is supposed to switch the setting from partial to complete"
        n542 = Array Size(array=w998) -> (size(s)=w1007:i32)
        n543 = Decrement(x=w1007) -> (x-1=w999:i32)
        n544 = Index Array(array=w998, index=w999) -> (element=w1002:T11)
        n545 = Unbundle By Name(w1002) -> ("SHOT STATUS"=w1006:u16)
        n546 = Equal To 0?(x=w1006) -> (x = 0?=w1005:bool)
        n547 = Select(t=u16 1, s=w1005, f=u16 0) -> (s? t:f=w1001:u16)
        n548 = local write "Current/sthotstatus"(w1001) -> ()
        n549 = Bundle By Name(cluster=w1002, "SHOT STATUS"=w1001) -> (w1000:T11)
        n550 = Replace Array Subset(array=w998, new element=w1000, index=w999) -> (w997:T1)
        n551 = stacked-sequence {
          tunnel: w1001 -> [_]
          tunnel: w997 -> [w1009]
          frame #0 {
            n552 = local write "SHOTS"(w1009) -> ()
            n553 = call "Sort Shots.vi"("shot array"=w1009) -> ("shotTable OUT"=w1010:string[][])
            n554 = local write "Table of Shots"(w1010) -> ()
          }
        }
      }
      frame 5 {
        (unwired) u8 0 ("Disabled")
        w1046 = -1 ("index of element")
        # "This section accepts new data"
        # "Shot Order"
        n555 = local read "Impact/speed"() -> (w1025:dbl)
        n556 = local read "residual/speed"() -> (w1024:dbl)
        n557 = local read "BACKFACE DIAMETER"() -> (w1039:dbl)
        n558 = local read "Corrected Residual"() -> (w1033:dbl)
        n559 = local read "Corrected Impact"() -> (w1031:dbl)
        n560 = local write "Accept Data"(FALSE) -> ()
        n561 = local read "metric conversion"() -> (w1016:dbl)
        n562 = local read "SHOT STATUS"() -> (w1038:u16)
        n563 = Format Date/Time String(time format string (%c)="%x   %H:%M:%S") -> (date/time string=w1045:string)  [unwired: 2 in]
        "SUBMIT DATE/TIME" <- w1045
        n564 = local read "Current/impact/speed"() -> (w1030:dbl)
        n565 = local read "BACKFACE DEPTH"() -> (w1026:dbl)
        n566 = local read "Current/residual/speed"() -> (w1032:dbl)
        n567 = Multiply(x=w1025, y=w1016) -> (x*y=w1018:dbl)
        n568 = Multiply(x=w1016, y=w1024) -> (x*y=w1017:dbl)
        n569 = Multiply(x=w1018, y=w1018) -> (x*y=w1023:dbl)
        n570 = Multiply(x=w1017, y=w1017) -> (x*y=w1022:dbl)
        n571 = Subtract(x=w1023, y=w1022) -> (x-y=w1020:dbl)
        n572 = Array Size(array=w1028) -> (size(s)=w1037:i32)
        n573 = Compound Arithmetic op=MULTIPLY("Projectile Mass", w1020, 0.0005 ("Input")) -> (w1015:dbl)
        n574 = local read "Corrected Redundant"() -> (w1012:dbl)
        n575 = Increment(x=w1037) -> (x+1=w1027:i32)
        n576 = Index Array(array=w1028) -> (element=w1041:T11)  [unwired: 1 in]
        n577 = Bundle By Name(cluster=w1041, "IMPACT VELOCITY"=w1025, "RESIDUAL  VELOCITY"=w1024, "Shot Description"="Shot Decription", "Powder Loading"="Powder Loading", "Barrel Temperature"="Barrel Temp", "TIME / DATE"=w1045, "shot order"=w1027, "SHOT STATUS"=w1038, "BackFace\nDepth"=w1026, "BackFace\nDiameter"=w1039, "Shot Angle"="Shot Angle", "Uncorrected Impact"=w1030, "Corrected Impact"=w1031, "Uncorrected Residual"=w1032, "Corrected residual"=w1033, "Projectile Mass"="Projectile Mass", "Energy Loss (J)"=w1015, "Red Vel"=w1012) -> (w1034:T11)
        n578 = Build Array (concatenate)(w1028, w1034) -> (w1013:T1)
        n579 = call "Sort Shots.vi"("shot array"=w1013) -> ("shotTable OUT"=w1014:string[][])
        n580 = local write "SHOTS"(w1013) -> ()
        n581 = local write "Table of Shots"(w1014) -> ()
        n582 = property on="Reject shot" class="Bool"("Disabled"=u8 0) -> ()  [unwired: 2 in, 2 out]
      }
      frame 6 {
        w1054 = -1
        # "This section will reset range"
        n583 = Concatenate Strings(w1050, "6|") -> (w1049:string)
        n584 = case shown="2" "Data Source" {
          tunnel: w1049 -> [_ _ w1062]
          tunnel: [w1055 w1056 w1058] -> w1048
          tunnel: w1047 -> [w1055 w1056 w1057]
          frame 0, Default {
          }
          frame 1 {
          }
          frame 2 {
            w1067 = u32 22 items=["NI-DAQ version", "device name", "base address", "data transfer mode for analog input", "data transfer mode for analog output group 1", "data transfer mode for analog output group 2", "data transfer mode for GPCTR 0", "data transfer mode for GPCTR 1", "data transfer mode for digital I/O group 1", "data transfer mode for digital I/O group 2", "device type code", "DMA A level", "DMA B level", "DMA C level", "interrupt A level", "interrupt B level", "reserved", "lpt device mode", "DAQCard-700 counter 1 source", "interrupt generation mode", "device state during suspend mode", "computer name", "serial number", "counter type", "Scarab A Memory Size", "Scarab B Memory Size"] ("information type")
            w1066 = u32 1  # device
            # "Screens"
            n585 = Concatenate Strings(w1062, "2|") -> (w1061:string)
            n586 = call "Get DAQ Device Information.vi"("information type"=w1067, "task ID or device"=w1066) -> ("error out"=w1060:errorcluster, "information string"=w1065:string)  [unwired: 7 in, 1 out]
            n587 = disable-structure shown="Disabled" {
              disable-tunnel: w1061 -> [w1073 _]
              disable-tunnel: w1060 -> [w1070 w1075]
              disable-tunnel: [w1069 w1075] -> w1059
              frame Disabled {
                n588 = Current VI's Path() -> (path=w1074:path)
                n589 = call "Where Am I (SubVI).vi"("TL Calling Location"=w1073, "Call VI path"=w1074) -> ("I'm here"=w1072:string)
                n590 = call "Error Check (SubVI).vi"("calling VI"=w1072, "tag #"=0, "error IN"=w1070) -> ("error OUT"=w1069:errorcluster)  [unwired: 2 in]
              }
              frame Enabled {
                # "Debug code is disabled"
              }
            }
            n591 = Unbundle By Name(w1060) -> ("status"=w1068:bool)
            n592 = case shown="False" w1068 {
              tunnel: w1065 -> [w1084 _]
              tunnel: [w1084 "DEVICE NOT READY!" ("information string")] -> w1064
              tunnel: w1059 -> [w1083 _]
              tunnel: [w1076 w1089] -> w1058
              tunnel: w1057 -> [_ w1089]
              frame False {
                # "assign task IDs to counters"
                n593 = call "Config Counter to Measure Two Edge Separation.vi"("error IN"=w1083, "Counter"="Impact Timer", "device"="DAQ Card") -> ("error out"=w1086:errorcluster, "task ID out"=w1079:u32)  [unwired: 1 in]
                "impact/ID" <- w1079
                n594 = call "Config Counter to Measure Two Edge Separation.vi"("error IN"=w1086, "Counter"="Residual  Timer", "device"="DAQ Card") -> ("error out"=w1088:errorcluster, "task ID out"=w1077:u32)  [unwired: 1 in]
                "residual/ID" <- w1077
                n595 = call "Config Counter to Measure Two Edge Separation.vi"("error IN"=w1088, "Counter"="Redundant Timer", "device"="DAQ Card") -> ("error out"=w1087:errorcluster, "task ID out"=w1078:u32)  [unwired: 1 in]
                "Red/ID" <- w1078
                n596 = Bundle("task ID out"=w1079, "task ID out"=w1078, "task ID out"=w1077) -> (w1076:T15)  [unwired: 1 in]
                n597 = call <vilib>:"Simple Error Handler.vi"("error in (no error)"=w1087) -> ()  [unwired: 4 in, 5 out]
              }
              frame True {
                w1092 = u16 0 items=["Simulated", "Radar", "Screens"] ("Data Source")
                n598 = local write "Data Source"(w1092) -> ()
                n599 = One Button Dialog(message="Error initializing Timer board.  Switching to simulation") -> ()  [unwired: 1 in, 1 out]
              }
            }
            "Device S/N" <- w1064
          }
        }
        n600 = local write "SUBMIT DATE/TIME"("") -> ()
      }
      frame 7 {
        w1098 = -1
        # "This section unaccepts new data  OR deletes the currently accessed previous shot"
        n601 = local read "Delete Button"() -> (w1097:bool)
        n602 = case shown="True" w1097 {
          tunnel: w1096 -> [w1101 w1113]
          tunnel: [w1102 w1114] -> w1094
          frame False {
            n603 = Array Size(array=w1101) -> (size(s)=w1099:i32)
            n604 = local write "SUBMIT DATE/TIME"("") -> ()
            n605 = while {
              tunnel: [w1105] -> w1100
              tunnel: w1099 -> [w1107]
              tunnel: w1101 -> [w1109] mode=indexing
              i -> [w1105]
              stop <- w1108 stop-if-true
              n606 = Unbundle By Name(w1109) -> ("shot order"=w1106:i32)
              n607 = Equal?(x=w1106, y=w1107) -> (x = y?=w1108:bool)
            }
            n608 = Delete From Array "Delete From Array"(array=w1101, index=w1100) -> (array with subset deleted=w1102:T1)  [unwired: 1 in, 1 out]
            n609 = property on="Reject shot" class="Bool"("Disabled"=u8 2) -> ()  [unwired: 2 in, 2 out]
          }
          frame True {
            n610 = property on="SHOTS" class="Arr (strict)"() -> ("Index Values"=w1122:u32[])  [unwired: 2 in, 2 out]
            n611 = local write "Delete Button"(FALSE) -> ()
            n612 = Index Array(array=w1122, index=0 ("Index")) -> (element=w1112:u32)
            n613 = Index Array(array=w1113, index=w1112) -> (element=w1111:T11)
            n614 = Unbundle By Name(w1111) -> ("shot order"=w1110:i32)
            n615 = Format Into String(format string="The currently displayed Shot, #%d", w1110) -> (resulting string=w1119:string)  [unwired: 2 in, 1 out]
            n616 = Concatenate Strings(w1119, ", will be deleted.  IT CANNOT RECOVERED!  Do you want to DELETE the shot?" ("message")) -> (w1118:string)
            n617 = Two Button Dialog(message=w1118, 1:"NO I do NOT want to delete.  Cancel Request" ("F button name (\"Cancel\")"), 2:"YES I want to delete the shot" ("T button name (\"OK\")")) -> (T button?=w1125:bool)
            n618 = case shown="True" w1125 {
              tunnel: w1113 -> [w1138 w1141]
              tunnel: [w1138 w1144] -> w1116
              tunnel: w1112 -> [_ w1143]
              tunnel: [10000 ("shot order") w1142] -> w1115
              frame False {
              }
              frame True {
                n619 = stacked-sequence {
                  tunnel: w1143 -> [w1145]
                  tunnel: [w1147] -> w1142
                  tunnel: w1141 -> [w1146]
                  tunnel: [w1146] -> w1140
                  tunnel: [w1145] -> w1139
                  frame #0 {
                    n620 = Index Array(array=w1146, index=w1145) -> (element=w1148:T11)
                    n621 = Unbundle By Name(w1148) -> ("shot order"=w1147:i32)
                  }
                }
                n622 = Delete From Array(array=w1140, index=w1139) -> (array with subset deleted=w1144:T1)  [unwired: 1 in, 1 out]
              }
            }
            n623 = for {
              tunnel: [w1132] -> w1114 mode=indexing
              tunnel: w1116 -> [w1127] mode=indexing
              tunnel: w1115 -> [w1131]
              n624 = Unbundle By Name(w1127) -> ("shot order"=w1129:i32)
              n625 = Decrement(x=w1129) -> (x-1=w1128:i32)
              n626 = Greater?(x=w1129, y=w1131) -> (0:w1130:bool)
              n627 = case shown="True" w1130 {
                tunnel: w1128 -> [_ w1135]
                tunnel: w1127 -> [w1133 w1136]
                tunnel: [w1133 w1134] -> w1132
                frame False {
                }
                frame True {
                  n628 = Bundle By Name(cluster=w1136, "shot order"=w1135) -> (w1134:T11)
                }
              }
            }
          }
        }
        n629 = call "Sort Shots.vi"("shot array"=w1094) -> ("shotTable OUT"=w1095:string[][])
        n630 = local write "Table of Shots"(w1095) -> ()
        n631 = local write "SHOTS"(w1094) -> ()
      }
      frame 8 {
        w1151 = 0.0 ("Input 1")
        w1161 = "TBD" ("Input 2")
        w1173 = TRUE  # append on new line? (F)
        w1186 = TRUE  # append on new line? (F)
        w1211 = FALSE  # show grid lines
        w1221 = -1 ("index of element")
        # "This section prepares a Contact Shot report"
        # "add graph to 3rd box"
        n632 = call <vilib>:"New Report.vi"("report type"=enum16{"Standard Report", "HTML"}."HTML") -> ("report out"=w1213:refnum<class "NI_report.lvclass">, "error out"=w1212:errorcluster)  [unwired: 13 in]
        n633 = call-dynamic "Set Report Font.vi"("report in"=w1213, "text options"=T10 {"Italic"=enum."Italic Unchanged", "Strike Through"=enum."Strike Through Unchanged", "Underline"=enum."Underline Unchanged", "Bold"=enum."Bold On"}, "font settings"=T9 {"Charset (-1)"=-1, "Weight (-1)"=-1, "Name"="Arial", "Size"="4 "}, "error in (no error)"=w1212) -> ("report out"=w1196:refnum<class "NI_report.lvclass">, "error out"=w1197:errorcluster)  [unwired: 9 in, 1 out]
        n634 = call-dynamic "Set Report Header Text.vi"("report in"=w1196, "center header text"="PBBA Ballistic CONTACT SHOT Report ", "error in (no error)"=w1197, "HTML header size"=enum16{"H1", "H2", "H3", "H4", "H5", "H6", "H7"}."H1") -> ("report out"=w1199:refnum<class "NI_report.lvclass">, "error out"=w1200:errorcluster)  [unwired: 10 in]
        n635 = call-dynamic "Set Report Font.vi"("report in"=w1199, "text options"=T10 {"Italic"=enum."Italic Unchanged", "Strike Through"=enum."Strike Through Unchanged", "Underline"=enum."Underline Unchanged", "Bold"=enum."Bold Off"}, "font settings"=T9 {"Charset (-1)"=-1, "Weight (-1)"=-1, "Name"="Arial", "Size"="1"}, "error in (no error)"=w1200) -> ("report out"=w1184:refnum<class "NI_report.lvclass">, "error out"=w1185:errorcluster)  [unwired: 9 in, 1 out]
        n636 = call-poly <vilib>:"Append Report Text.vi"("report in"=w1184, "text"="Disclosure on Ballistic and Stab Test Data<newline>The attached ballistic test data was generated by PBBA and corresponds to PBBA's current knowledge on the performance of the subject test panels against certain ballistic threats.  This information is offered solely to provide possible suggestions for your own experimentation and validation.  It is not intended as a substitute for your own testing or any testing you may need to submit for a bid package, you should undertake your own testing whether you do so yourself with the supplier of the materials to be tested or with an independent, third party, certified testing facility and the supplier of the materials to be tested (i.e., the fabric weaver).  PBBA makes no warranties, and assumes no liabilities in connection with any use of the information supplied with this disclosure statement.", "error in (no error)"=w1185) -> ("report out"=w1183:refnum<class "NI_report.lvclass">, "error out"=w1181:errorcluster)  [unwired: 9 in, 2 out]
        n637 = local read "Sample ID"() -> (w1150:string)
        n638 = call-dynamic "Set Report Font.vi"("report in"=w1183, "text options"=T10 {"Italic"=enum."Italic Unchanged", "Strike Through"=enum."Strike Through Unchanged", "Underline"=enum."Underline Unchanged", "Bold"=enum."Bold Unchanged"}, "font settings"=T9 {"Charset (-1)"=-1, "Weight (-1)"=-1, "Name"="Arial", "Size"="3 "}, "error in (no error)"=w1181) -> ("report out"=w1182:refnum<class "NI_report.lvclass">, "error out"=w1180:errorcluster)  [unwired: 9 in, 1 out]
        n639 = call-dynamic "New Report Line.vi"("report in"=w1182, "error in (no error)"=w1180) -> ("report out"=w1214:refnum<class "NI_report.lvclass">, "error out"=w1215:errorcluster)  [unwired: 12 in]
        n640 = call-dynamic "New Report Line.vi"("report in"=w1214, "error in (no error)"=w1215) -> ("report out"=w1188:refnum<class "NI_report.lvclass">, "error out"=w1187:errorcluster)  [unwired: 12 in]
        n641 = Format Into String(format string="<table border=\"0\" cellspacing=\"6\"><tr><td align=\"left\"><b>Fabric Parameters</b></td><td>&nbsp;</td><td>&nbsp;</td><td align=\"left\"><b>Test Parameters</b></td><td>&nbsp;</td></tr><tr><td align=\"right\">Sample ID: </td><td align=\"left\">%s</td><td>&nbsp;</td><td align=\"right\">Method: </td><td align=\"left\">V50</td></tr><tr><td align=\"right\">Areal Density: </td><td align=\"left\">%.3f</td><td>&nbsp;</td><td align=\"right\">Threat: </td><td align=\"left\">%s</td></tr><tr><td align=\"right\">Manufacturer: </td><td align=\"left\">%s</td><td>&nbsp;</td><td align=\"right\">Room Temperature: </td><td align=\"left\">%.0f</td></tr><tr><td align=\"right\">Group Data: </td><td align=\"left\">%s</td><td>&nbsp;</td><td align=\"right\">Correction Factor: </td><td align=\"left\">%0.4f</td></tr><tr><td align=\"right\">Projectile Weight: </td><td align=\"left\">%0.3f</td><td>&nbsp;</td><td align=\"right\">Panel Backing: </td><td align=\"left\">%s</td></tr><tr><td align=\"right\">Powder Type: </td><td align=\"left\">%s</td><td>&nbsp;</td><td align=\"right\">Shot Angle: </td><td align=\"left\">%.0f</td></tr><tr><td align=\"right\">Test Conditions: </td><td align=\"left\">%s</td><td>&nbsp;</td><td align=\"right\">Room Humidity: </td><td align=\"left\">%.0f</td></tr><tr><td align=\"right\">Panel Weight: </td><td align=\"left\">%.4f</td><td>&nbsp;</td><td>&nbsp;</td></tr><tr><td align=\"right\">Descripton: </td><td align=\"left\">%s</td><td>&nbsp;</td><td>&nbsp;</td></tr></table>", w1150, w1151, w1161, w1161, w1151, w1161, w1151, w1151, w1161, w1161, w1151, w1161, w1151, w1151, w1161) -> (resulting string=w1172:string)  [unwired: 2 in, 1 out]
        n642 = call-poly <vilib>:"Append Report Text.vi"("report in"=w1188, "text"=w1172, "append on new line? (F)"=w1186, "error in (no error)"=w1187) -> ("report out"=w1167:refnum<class "NI_report.lvclass">, "error out"=w1168:errorcluster)  [unwired: 8 in, 2 out]
        n643 = call-dynamic "New Report Line.vi"("report in"=w1167, "error in (no error)"=w1168) -> ("report out"=w1208:refnum<class "NI_report.lvclass">, "error out"=w1209:errorcluster)  [unwired: 12 in]
        n644 = call-dynamic "New Report Line.vi"("report in"=w1208, "error in (no error)"=w1209) -> ("report out"=w1207:refnum<class "NI_report.lvclass">, "error out"=w1206:errorcluster)  [unwired: 12 in]
        n645 = call-poly <vilib>:"Append Table to Report.vi"("report in"=w1207, "column width (1)"=1.1, "text data"=string[][] [["TBD"]], "error in (no error)"=w1206, "show grid lines"=w1211) -> ("report out"=w1174:refnum<class "NI_report.lvclass">, "error out"=w1178:errorcluster)  [unwired: 7 in, 2 out]
        n646 = call-dynamic "Set Report Font.vi"("report in"=w1174, "text options"=T10 {"Italic"=enum."Italic Unchanged", "Strike Through"=enum."Strike Through Unchanged", "Underline"=enum."Underline On", "Bold"=enum."Bold Off"}, "font settings"=T9 {"Charset (-1)"=-1, "Weight (-1)"=-1, "Name"="Arial", "Size"="3 "}, "error in (no error)"=w1178) -> ("report out"=w1175:refnum<class "NI_report.lvclass">, "error out"=w1176:errorcluster)  [unwired: 9 in, 1 out]
        n647 = call-dynamic "New Report Line.vi"("report in"=w1175, "error in (no error)"=w1176) -> ("report out"=w1205:refnum<class "NI_report.lvclass">, "error out"=w1204:errorcluster)  [unwired: 12 in]
        n648 = call-poly <vilib>:"Append Report Text.vi"("report in"=w1205, "append on new line? (F)"=w1173, "error in (no error)"=w1204) -> ("report out"=w1165:refnum<class "NI_report.lvclass">, "error out"=w1164:errorcluster)  [unwired: 9 in, 2 out]
        n649 = control-ref of="Shot Graph"() -> (w1157:refnum<vi>)
        n650 = local read "Sample ID"() -> (w1152:string)
        n651 = call-dynamic "Append Control Image to Report.vi"("report in"=w1165, "image file type (.jpg)"=enum16{".jpg", ".png"}.".jpg" ("image file type(.png)"), "ctrl reference"=w1157, "description"="Graph of Test Results" ("control name"), "error in (no error)"=w1164) -> ("report out"=w1162:refnum<class "NI_report.lvclass">, "error out"=w1163:errorcluster)  [unwired: 7 in, 2 out]
        n652 = local read "Report Path"() -> (w1153:path)
        n653 = Format Value(format string="SHOT %s.html  " ("string (\"\")"), value (0)=w1152) -> (output string=w1191:string)  [unwired: 1 in]
        n654 = call-dynamic "Set Report Footer Text.vi"("report in"=w1162, "error in (no error)"=w1163) -> ("report out"=w1201:refnum<class "NI_report.lvclass">, "error out"=w1202:errorcluster)  [unwired: 12 in]
        n655 = Build Path(base path=w1153, name or relative path=w1191) -> (appended path=w1189:path)
        n656 = call-dynamic "Get Report Type.vi"("report in"=w1201, "error in (no error)"=w1202) -> ("report out"=w1217:refnum<class "NI_report.lvclass">, "report type"=w1216:T14, "error out"=w1220:errorcluster)  [unwired: 11 in]
        n657 = case shown="\"Standard Report\", Default" w1216 {
          tunnel: w1217 -> [w1227 w1232]
          tunnel: [w1226 w1231] -> w1218
          tunnel: [w1225 w1230] -> w1219
          tunnel: w1220 -> [w1224 w1229]
          tunnel: w1189 -> [w1223 w1228]
          tunnel: [w1223 w1228] -> _
          frame "Standard Report", Default {
            n658 = call-dynamic "Print Report.vi"("report in"=w1227, "error in (no error)"=w1224) -> ("report out"=w1226:refnum<class "NI_report.lvclass">, "error out"=w1225:errorcluster)  [unwired: 12 in]
          }
          frame "HTML" {
            n659 = call-dynamic "Save Report to File.vi"("report in"=w1232, "report file path"=w1228, "error in (no error)"=w1229) -> ("report out"=w1231:refnum<class "NI_report.lvclass">, "error out"=w1230:errorcluster)  [unwired: 11 in]
          }
        }
        n660 = call-dynamic "Dispose Report.vi"("report in"=w1218, "error in (no error)"=w1219) -> ("error out"=w1169:errorcluster)  [unwired: 13 in]
        n661 = call <vilib>:"Simple Error Handler.vi"("error in (no error)"=w1169) -> ("error out"=w1170:errorcluster)  [unwired: 4 in, 4 out]
        n662 = case shown="No Error" w1170 {
          frame No Error {
            n663 = One Button Dialog(message="A CONTACT SHOT Report is ready.") -> ()  [unwired: 1 in, 1 out]
          }
          frame Error {
          }
        }
      }
    }
    n664 = Wait (ms)(milliseconds to wait=u32 20 ("millisecond timer value")) -> ()  [unwired: 1 out]
  }
